vi "main 0.9.6.testing.vi"() -> ()   [LabVIEW 2015]
uses:
  subvi/PHOIBOS/DEFINITIONS/DEF_dev_state.ctl
  subvi/PHOIBOS/DEFINITIONS/DEF_dev_type.ctl
  <vilib>/Analysis/1siggen.llb/Ramp Pattern by Samples.vi
  <vilib>/DAQmx/read.llb/DAQmx Read (Digital Bool 1Line 1Point).vi
  <vilib>/Utility/file.llb/Write Delimited Spreadsheet (DBL).vi
  <vilib>/Utility/file.llb/Read Delimited Spreadsheet (string).vi
  <vilib>/DAQmx/create/channels.llb/DAQmx Create Channel (DI-Digital Input).vi
  <vilib>/DAQmx/miscellaneous.llb/DAQmx Fill In Error Info.vi
  subvi/Newport ESP301/Newport ESP301.lvlib
  subvi/sp_manip.llb/sp_manip_lib.lvlib
  subvi/sp_manip.llb/tcp_gateway.lvlib
  <vilib>/Analysis/NI_AALBase.lvlib
panel:
  in  "Enable Chopping":bool
  out "Pump Laser":bool
  out "Pics L":i32
  out "Pics NL":i32
  out "sideimg 2":dbl[][](graph)
  in  "Frame trigger \n(High Performance and QE only)":u16=1
  in  "Operating mode\nHP & QE / HS & DiCam Pro":u32
  out "Waveform Chart":dbl(graph)
  out "G2 X":cluster{dbl[], "Ramp Pattern":dbl[]}(graph)={array[344 elements], "Ramp Pattern"=[5593.0, 5541.0, 5578.0, 5573.0, 5542.0, 5582.0, 5523.0, 5570.0, 5578.0, 5560.0, 5581.0, 5542.0, 5577.0, 5517.0, 5599.0, 5558.0, 5549.0, 5571.0, 5527.0, 5574.0, 5565.0, 5561.0, 5570.0, 5531.0, 5576.0, 5531.0, 5576.0, 5554.0, 5523.0, 5573.0, 5536.0, 5555.0, 5539.0, 5549.0, 5543.0, 5541.0, 5581.0, 5523.0, 5548.0, 5528.0, 5558.0, 5565.0, 5537.0, 5556.0, 5521.0, 5538.0, 5549.0, 5532.0, 5562.0, 5512.0, 5555.0, 5549.0, 5536.0, 5542.0, 5511.0, 5567.0, 5526.0, 5549.0, 5545.0, 5543.0, 5562.0, 5518.0, 5561.0, 5490.0, 5542.0, 5522.0, 5529.0, 5542.0, 5521.0, 5556.0, 5511.0, 5541.0, 5534.0, 5512.0, 5569.0, 5525.0, 5547.0, 5507.0, 5533.0, 5533.0, 5501.0, 5555.0, 5497.0, 5517.0, 5526.0, 5519.0, 5565.0, 5503.0, 5548.0, 5496.0, 5544.0, 5523.0, 5534.0, 5533.0, 5501.0, 5529.0, 5494.0, 5523.0, 5526.0, 5519.0, 5539.0, 5493.0, 5508.0, 5532.0, 5504.0, 5546.0, 5540.0, 5550.0, 5488.0, 5556.0, 5535.0, 5510.0, 5535.0, 5515.0, 5543.0, 5475.0, 5538.0, 5528.0, 5504.0, 5523.0, 5502.0, 5535.0, 5473.0, 5503.0, 5501.0, 5531.0, 5525.0, 5490.0, 5524.0, 5484.0, 5520.0, 5506.0, 5492.0, 5516.0, 5477.0, 5511.0, 5487.0, 5509.0, 5496.0, 5467.0, 5538.0, 5494.0, 5512.0, 5497.0, 5498.0, 5526.0, 5482.0, 5506.0, 5466.0, 5522.0, 5489.0, 5512.0, 5518.0, 5475.0, 5547.0, 5480.0, 5569.0, 5504.0, 5485.0, 5528.0, 5506.0, 5529.0, 5468.0, 5524.0, 5507.0, 5518.0, 5511.0, 5471.0, 5525.0, 5480.0, 5482.0, 5510.0, 5506.0, 5522.0, 5475.0, 5540.0, 5477.0, 5511.0, 5514.0, 5500.0, 5497.0, 5484.0, 5536.0, 5476.0, 5485.0, 5527.0, 5509.0, 5529.0, 5495.0, 5504.0, 5496.0, 5519.0, 5512.0, 5469.0, 5506.0, 5465.0, 5502.0, 5481.0, 5508.0, 5519.0, 5499.0, 5515.0, 5476.0, 5496.0, 5502.0, 5499.0, 5494.0, 5477.0, 5541.0, 5477.0, 5512.0, 5497.0, 5472.0, 5511.0, 5471.0, 5503.0, 5507.0, 5504.0, 5477.0, 5479.0, 5508.0, 5481.0, 5522.0, 5517.0, 5516.0, 5505.0, 5502.0, 5491.0, 5481.0, 5512.0, 5484.0, 5500.0, 5478.0, 5493.0, 5529.0, 5492.0, 5518.0, 5471.0, 5518.0, 5490.0, 5513.0, 5497.0, 5488.0, 5517.0, 5477.0, 5524.0, 5464.0, 5495.0, 5514.0, 5495.0, 5522.0, 5477.0, 5490.0, 5535.0, 5489.0, 5491.0, 5491.0, 5515.0, 5473.0, 5504.0, 5505.0, 5515.0, 5510.0, 5473.0, 5521.0, 5475.0, 5537.0, 5499.0, 5505.0, 5509.0, 5460.0, 5509.0, 5473.0, 5489.0, 5500.0, 5464.0, 5522.0, 5471.0, 5528.0, 5475.0, 5502.0, 5494.0, 5511.0, 5516.0, 5486.0, 5528.0, 5471.0, 5492.0, 5477.0, 5491.0, 5531.0, 5486.0, 5549.0, 5498.0, 5524.0, 5482.0, 5495.0, 5505.0, 5476.0, 5512.0, 5444.0, 5512.0, 5498.0, 5471.0, 5489.0, 5462.0, 5502.0, 5459.0, 5503.0, 5489.0, 5493.0, 5498.0, 5461.0, 5505.0, 5495.0, 5503.0, 5459.0, 5501.0, 5515.0, 5459.0, 5510.0, 5469.0, 5504.0, 5499.0, 5505.0, 5524.0, 5477.0, 5527.0, 5477.0, 5475.0, 5495.0, 5482.0, 5514.0, 5481.0, 5499.0, 5481.0, 5482.0, 5498.0, 5460.0, 5469.0, 5471.0, 5519.0, 5495.0, 5485.0]}
  in  "reset every n pics":bool
  in  "pics2avg":i32=50
  in  "abort acq.":bool
  out "G2 Y":cluster{dbl[], "Ramp Pattern":dbl[]}(graph)={[5738.0, 5692.0, 5562.0, 5630.0, 5633.0, 5616.0, 5523.0, 5622.0, 5406.0, 5598.0, 5416.0, 5403.0, 5579.0, 5325.0, 5504.0, 5402.0, 5538.0, 5568.0, 5460.0, 5494.0, 5367.0, 5597.0, 5434.0, 5448.0, 5339.0, 5434.0, 5460.0, 5482.0, 5646.0, 5720.0, 5704.0, 5628.0, 5672.0, 5511.0, 5420.0, 5539.0, 5543.0, 5421.0, 5486.0, 5508.0, 5537.0, 5586.0, 5460.0, 5547.0, 5433.0, 5488.0, 5552.0, 5538.0, 5528.0, 5482.0, 5406.0, 5458.0, 5644.0, 5485.0, 5443.0, 5485.0, 5385.0, 5413.0, 5472.0, 5571.0, 5640.0, 5602.0, 5462.0, 5477.0, 5408.0, 5396.0, 5445.0, 5638.0, 5383.0, 5571.0, 5372.0, 5519.0, 5426.0, 5462.0, 5481.0, 5626.0, 5326.0, 5458.0, 5471.0, 5366.0, 5394.0, 5363.0, 5551.0, 5596.0, 5452.0, 5470.0, 5600.0, 5533.0, 5573.0, 5544.0, 5671.0, 5595.0, 5423.0, 5550.0, 5557.0, 5416.0, 5404.0, 5478.0, 5448.0, 5512.0, 5505.0, 5575.0, 5434.0, 5436.0, 5600.0, 5487.0, 5607.0, 5463.0, 5606.0, 5540.0, 5521.0, 5581.0, 5472.0, 5555.0, 5576.0, 5612.0, 5529.0, 5473.0, 5454.0, 5455.0, 5500.0, 5650.0, 5451.0, 5445.0, 5423.0, 5376.0, 5389.0, 5491.0, 5536.0, 5525.0, 5440.0, 5707.0, 5414.0, 5532.0, 5400.0, 5668.0, 5706.0, 5515.0, 5431.0, 5400.0, 5439.0, 5471.0, 5627.0, 5691.0, 5569.0, 5718.0, 5614.0, 5523.0, 5436.0, 5432.0, 5419.0, 5516.0, 5469.0, 5467.0, 5530.0, 5598.0, 5501.0, 5476.0, 5457.0, 5460.0, 5606.0, 5456.0, 5429.0, 5586.0, 5504.0, 5546.0, 5516.0, 5466.0, 5650.0, 5593.0, 5605.0, 5515.0, 5414.0, 5623.0, 5581.0, 5651.0, 5574.0, 5519.0, 5672.0, 5621.0, 5496.0, 5382.0, 5496.0, 5620.0, 5542.0, 5422.0, 5492.0, 5515.0, 5549.0, 5402.0, 5472.0, 5547.0, 5515.0, 5641.0, 5451.0, 5667.0, 5622.0, 5511.0, 5506.0, 5608.0, 5647.0, 5584.0, 5714.0, 5490.0, 5534.0, 5463.0, 5566.0, 5573.0, 5570.0, 5582.0, 5613.0, 5504.0, 5550.0, 5594.0, 5576.0, 5677.0, 5675.0, 5681.0, 5681.0, 5434.0, 5434.0, 5405.0, 5473.0, 5522.0, 5427.0, 5533.0, 5582.0, 5427.0, 5529.0, 5548.0, 5341.0, 5521.0, 5539.0, 5435.0, 5457.0, 5511.0, 5406.0, 5412.0, 5620.0, 5609.0, 5609.0, 5469.0, 5577.0, 5661.0, 5673.0, 5518.0, 5463.0, 5562.0, 5723.0, 5719.0, 5487.0, 5485.0, 5683.0, 5501.0, 5604.0, 5328.0], "Ramp Pattern"=[0.0, 1.003921568627451, 2.007843137254902, 3.011764705882353, 4.015686274509804, 5.019607843137255, 6.023529411764706, 7.027450980392157, 8.031372549019608, 9.035294117647059, 10.03921568627451, 11.04313725490196, 12.047058823529412, 13.050980392156863, 14.054901960784314, 15.058823529411764, 16.062745098039215, 17.066666666666666, 18.070588235294117, 19.07450980392157, 20.07843137254902, 21.08235294117647, 22.08627450980392, 23.090196078431372, 24.094117647058823, 25.098039215686274, 26.101960784313725, 27.105882352941176, 28.109803921568627, 29.113725490196078, 30.11764705882353, 31.12156862745098, 32.12549019607843, 33.129411764705885, 34.13333333333333, 35.13725490196079, 36.141176470588235, 37.14509803921569, 38.14901960784314, 39.15294117647059, 40.15686274509804, 41.16078431372549, 42.16470588235294, 43.168627450980395, 44.17254901960784, 45.1764705882353, 46.180392156862744, 47.1843137254902, 48.188235294117646, 49.1921568627451, 50.19607843137255, 51.2, 52.20392156862745, 53.207843137254905, 54.21176470588235, 55.21568627450981, 56.219607843137254, 57.22352941176471, 58.227450980392156, 59.23137254901961, 60.23529411764706, 61.23921568627451, 62.24313725490196, 63.247058823529414, 64.25098039215686, 65.25490196078431, 66.25882352941177, 67.26274509803922, 68.26666666666667, 69.27058823529411, 70.27450980392157, 71.27843137254902, 72.28235294117647, 73.28627450980392, 74.29019607843138, 75.29411764705883, 76.29803921568627, 77.30196078431372, 78.30588235294118, 79.30980392156863, 80.31372549019608, 81.31764705882352, 82.32156862745099, 83.32549019607843, 84.32941176470588, 85.33333333333333, 86.33725490196079, 87.34117647058824, 88.34509803921569, 89.34901960784313, 90.3529411764706, 91.35686274509804, 92.36078431372549, 93.36470588235294, 94.3686274509804, 95.37254901960785, 96.37647058823529, 97.38039215686274, 98.3843137254902, 99.38823529411765, 100.3921568627451, 101.39607843137254, 102.4, 103.40392156862745, 104.4078431372549, 105.41176470588235, 106.41568627450981, 107.41960784313726, 108.4235294117647, 109.42745098039215, 110.43137254901961, 111.43529411764706, 112.43921568627451, 113.44313725490196, 114.44705882352942, 115.45098039215686, 116.45490196078431, 117.45882352941176, 118.46274509803922, 119.46666666666667, 120.47058823529412, 121.47450980392156, 122.47843137254903, 123.48235294117647, 124.48627450980392, 125.49019607843137, 126.49411764705883, 127.49803921568628, 128.50196078431372, 129.50588235294117, 130.50980392156862, 131.51372549019607, 132.51764705882354, 133.521568627451, 134.52549019607844, 135.52941176470588, 136.53333333333333, 137.53725490196078, 138.54117647058823, 139.54509803921567, 140.54901960784315, 141.5529411764706, 142.55686274509804, 143.5607843137255, 144.56470588235294, 145.5686274509804, 146.57254901960783, 147.57647058823528, 148.58039215686276, 149.5843137254902, 150.58823529411765, 151.5921568627451, 152.59607843137255, 153.6, 154.60392156862744, 155.6078431372549, 156.61176470588236, 157.6156862745098, 158.61960784313726, 159.6235294117647, 160.62745098039215, 161.6313725490196, 162.63529411764705, 163.6392156862745, 164.64313725490197, 165.64705882352942, 166.65098039215687, 167.65490196078431, 168.65882352941176, 169.6627450980392, 170.66666666666666, 171.6705882352941, 172.67450980392158, 173.67843137254903, 174.68235294117648, 175.68627450980392, 176.69019607843137, 177.69411764705882, 178.69803921568626, 179.7019607843137, 180.7058823529412, 181.70980392156864, 182.71372549019608, 183.71764705882353, 184.72156862745098, 185.72549019607843, 186.72941176470587, 187.73333333333332, 188.7372549019608, 189.74117647058824, 190.7450980392157, 191.74901960784314, 192.75294117647059, 193.75686274509803, 194.76078431372548, 195.76470588235293, 196.7686274509804, 197.77254901960785, 198.7764705882353, 199.78039215686275, 200.7843137254902, 201.78823529411764, 202.7921568627451, 203.79607843137254, 204.8, 205.80392156862746, 206.8078431372549, 207.81176470588235, 208.8156862745098, 209.81960784313725, 210.8235294117647, 211.82745098039214, 212.83137254901962, 213.83529411764707, 214.8392156862745, 215.84313725490196, 216.8470588235294, 217.85098039215686, 218.8549019607843, 219.85882352941175, 220.86274509803923, 221.86666666666667, 222.87058823529412, 223.87450980392157, 224.87843137254902, 225.88235294117646, 226.8862745098039, 227.89019607843136, 228.89411764705883, 229.89803921568628, 230.90196078431373, 231.90588235294118, 232.90980392156862, 233.91372549019607, 234.91764705882352, 235.92156862745097, 236.92549019607844, 237.9294117647059, 238.93333333333334, 239.93725490196078, 240.94117647058823, 241.94509803921568, 242.94901960784313, 243.95294117647057, 244.95686274509805, 245.9607843137255, 246.96470588235294, 247.9686274509804, 248.97254901960784, 249.9764705882353, 250.98039215686273, 251.98431372549018, 252.98823529411766, 253.9921568627451, 254.99607843137255, 256.0]}
  out "ETA":timestamp=timestamp(3543843884.995538 s since 1904-01-01) format="%<%H:%M:%S>T"
  out "acq. imgs":i32=30
  out "snap_prog":dbl(slide)=1.0 scale=0.0..1.0
  in  "BasePath":path=path "C:/Users/femtolab_admin/Desktop"
  in  "cam_liveavg":bool caption="live average"
  out "cam_fps":dbl=20.079713544692744 caption="FPS" format="%.1g"
  out "sideimg":dbl[][](graph)
  in  "RunNumber":u16=77
  out "sum":dbl=4126991.0 format="%#.2g"
  out "max":dbl=54.0
  out "mainimg":dbl[][](graph)
  out "ESP_con?":bool=TRUE caption="ESP301"
  out "phoib_con?":bool caption="PHOIBOS"
  out "manip_con?":bool caption="manipulator"
  out "cam_con?":bool caption="camera"
  in  "main_close":bool
  in  "Tab Control":T1(tab)
  in  "manip_deltas":dbl[](array[numeric])=[0.0, 0.0, 0.0, 0.0, 10.0, 0.0] caption="delta" format="%#.5g"
  in  "aq.mode":enum32{"Radio Selection 1", "Radio Selection 2"}(radio)=enum."Radio Selection 2"
  in  "dark avg":i32=100
  in  "averages":i32=30 caption="N"
  in  "ESP_delta":dbl caption="relative [mm]"
  in  "ESP_-":bool
  in  "ESP_+":bool
  in  "ESP_go":bool
  in  "ESP_dest_t":dbl=250.17307139859977 caption="[fs]"
  in  "ESP_dest":dbl=31.304 caption="[mm]"
  in  "ESP_set_t0":bool
  in  "phoib_I_6s":dbl=3200.0
  in  "phoib_I_5s":dbl=1650.0
  in  "phoib_I_4s":dbl=4.558
  in  "phoib_I_3s":dbl=-7.0
  in  "phoib_I_2s":dbl=20.0
  in  "phoib_I_1s":dbl=22.0
  in  "phoib_standby":bool
  in  "phoib_set":bool
  out "phoib_I_6":dbl caption="Screen Voltage"
  out "phoib_I_5":dbl caption="Detctor Voltage"
  out "phoib_I_4":dbl caption="Work Function"
  out "phoib_I_3":dbl caption="Coil Current"
  out "phoib_I_2":dbl caption="Pass Energy"
  out "phoib_I_1":dbl caption="Kinetic Energy"
  out "Saved Positions":string[][](table)=[["ertwertwert", "-2.299945", "-2.030214", "38.900024", "50.000762", "0.000887", "-97.998082"], ["uztgugt", "-14.999451", "-13.638894", "442.380066", "13.998380", "-1.893758", "-76.305838"], ["asdf", "-14.999451", "-13.638894", "442.380066", "13.998380", "-1.893758", "-76.305838"], ["test3", "-14.999451", "-13.638894", "441.380066", "13.998380", "-1.893758", "-76.305838"]]
  in  "Save Pos":bool
  in  "Load":bool
  in  "Delete":bool
  in  "ManipRel +":bool
  in  "ManipRel -":bool
  in  "Move Abs":bool
  in  "stop manip":bool
  in  "dest":dbl[](array[numeric])=[-2.6172862113166087, -0.009888298846365134, 68.5008544921875, -46.36280498847848, 1.1073518432055398, -218.56360350415366] caption="destination" format="%#.5g"
  out "axis":string[](array[string])=["x", "y", "z", "polar", "tilt", "azimut"]
  out "pos":dbl[](array[numeric])=[-2.6172862113166087, -0.009888298846365134, 68.5008544921875, -46.363686276590336, 11.108982061941884, -218.56360350415366] caption="position" format="%.5f"
  in  "Mode":T2(ring)=enum."WideAngleMode"
  in  "VoltageRange":enum16{"3.5kV", "1.5kV", "400V", "100V", "10V"}(ring)=enum."400V"
  out "ESP_pos":dbl=31.4539 caption="Position"
  out "ESP_delay":dbl=1000.0251574040756 caption="Delay"
  out "ESP_t0":dbl=31.304 caption="Time Zero @"
  out "phoib_I_7":dbl caption="Conversion Voltage"
  in  "phoib_I_7s":dbl=-16.0
  in  "phoib_I_8s":dbl=0.0039
  in  "phoib_I_9s":dbl=0.0039
  out "phoib_I_8":dbl caption="FD1"
  out "phoib_I_9":dbl caption="FD2"
  in  "gain":bool
  in  "exposure [ms]":u32=1
  in  "binning":u16(ring)=2 items=["X 1", "X 2", "X 4", "X 8"]
  in  "cam_dark?":bool caption="subtract dark?"
  in  "cam_dark":bool
  in  "cam_saveimg":bool
  in  "e-size":u8
  in  "lower threshold":i32=-100
  in  "count?":bool
  in  "ROI Left":i32=1
  in  "ROI Right":i32=43
  in  "ROI Top":i32=1
  in  "ROI Bottom":i32=33
  out "moving?":bool[](array[boolean])
  in  "delscan_abort 2":bool
  in  "delscan_go 2":bool
  in  "delscan_finishIteration 2":bool
  out "del_ETA":timestamp=timestamp(3543843871.185777 s since 1904-01-01) format="%<%H:%M:%S>T"
  out "time / step":dbl=2.792118032773336
  out "duration [HH:MM:SS]":dbl=55.62603882380894 format="%<%H:%M:%S>t"
  out "disk [MB]":dbl=11.613000000000001
  out "RAM [MB]":dbl=2.765
  out "total steps":dbl=20.0
  out "delaypoints":dbl=5.0
  in  "generate delay table":bool
  in  "load delay table":bool
  in  "delay table [fs]":string[][](table)=[["-1000.000000"], ["-500.000000"], ["0.000000"], ["500.000000"], ["1000.000000"]]
  in  "delscan_iters":u32=4 caption="iterations"
  out "scangraph":T3(graph)
  in  "delscan_abort":bool
  out "delscan_progress":u32(slide)=5 scale=0.0..11.0
  in  "delscan_go":bool
  out "delscan_pos":dbl=31.453896228999998 caption="stage pos [mm]"
  in  "delscan_end":dbl=1000.0 caption="end [fs]"
  in  "delscan_stepsize":dbl=500.0 caption="stepsize [fs]"
  in  "delscan_start":dbl=-1000.0 caption="start [fs]"
  out "iteration":i32=5
  in  "delscan_finishIteration":bool
  in  "manip_scan_steps":u32=3
  in  "Optimize":bool
  in  "manip_scan_delta":dbl[](array[numeric])=[0.0, 0.0, 0.0, 0.0, 1.0, 0.0] caption="delta" format="%#.5g"
  out "delscan_progress 2":u32(slide)=2 scale=0.0..3.0
  in  "abort":bool
  in  "dev_bench":bool
  out "x/y":dbl
  out "1/x":dbl
  in  "stop":bool
  out "voltage out":dbl
  in  "manip_init":bool
  in  "manip_release":bool
  in  "phoib_init":bool
  in  "phoib_release":bool
  in  "ESP_init":bool
  in  "ESP_release":bool
  in  "ESP301 VISA":refnum<visa-resource-name>="COM8"
  in  "board number":i32
  in  "cam_init":bool
  in  "cam_release":bool
  out "cam_error":errorcluster
  out "phoib_error":errorcluster
  out "state":T4 items=["Off"=-1, "Standby"=0, "On"=1]
  in  "ESP Axis":i32=1 min=1 max=3
  out "error out":errorcluster
  out "error out 2":errorcluster={"status"=TRUE, "code"=1, "source"="TCP Write in sp_manip_lib.lvlib:sp_manip_disconnect.vi->main 0.9.1.vi"}
  # "0 = sequential\n1 = simultaneous"
  # "0 = internal\n1 = external rising\n2 = external falling"
  # "camera"
  # "analyzer"
  # "manipulator"
  # "aquisition"
  # "delay stage"
  # "Position"
  # "Destination"
  # "X\nY\nZ\npolar\ntilt\nazimut"
  # "camera"
  # "phoibos"
  # "ESP301"
  # "manipulator"
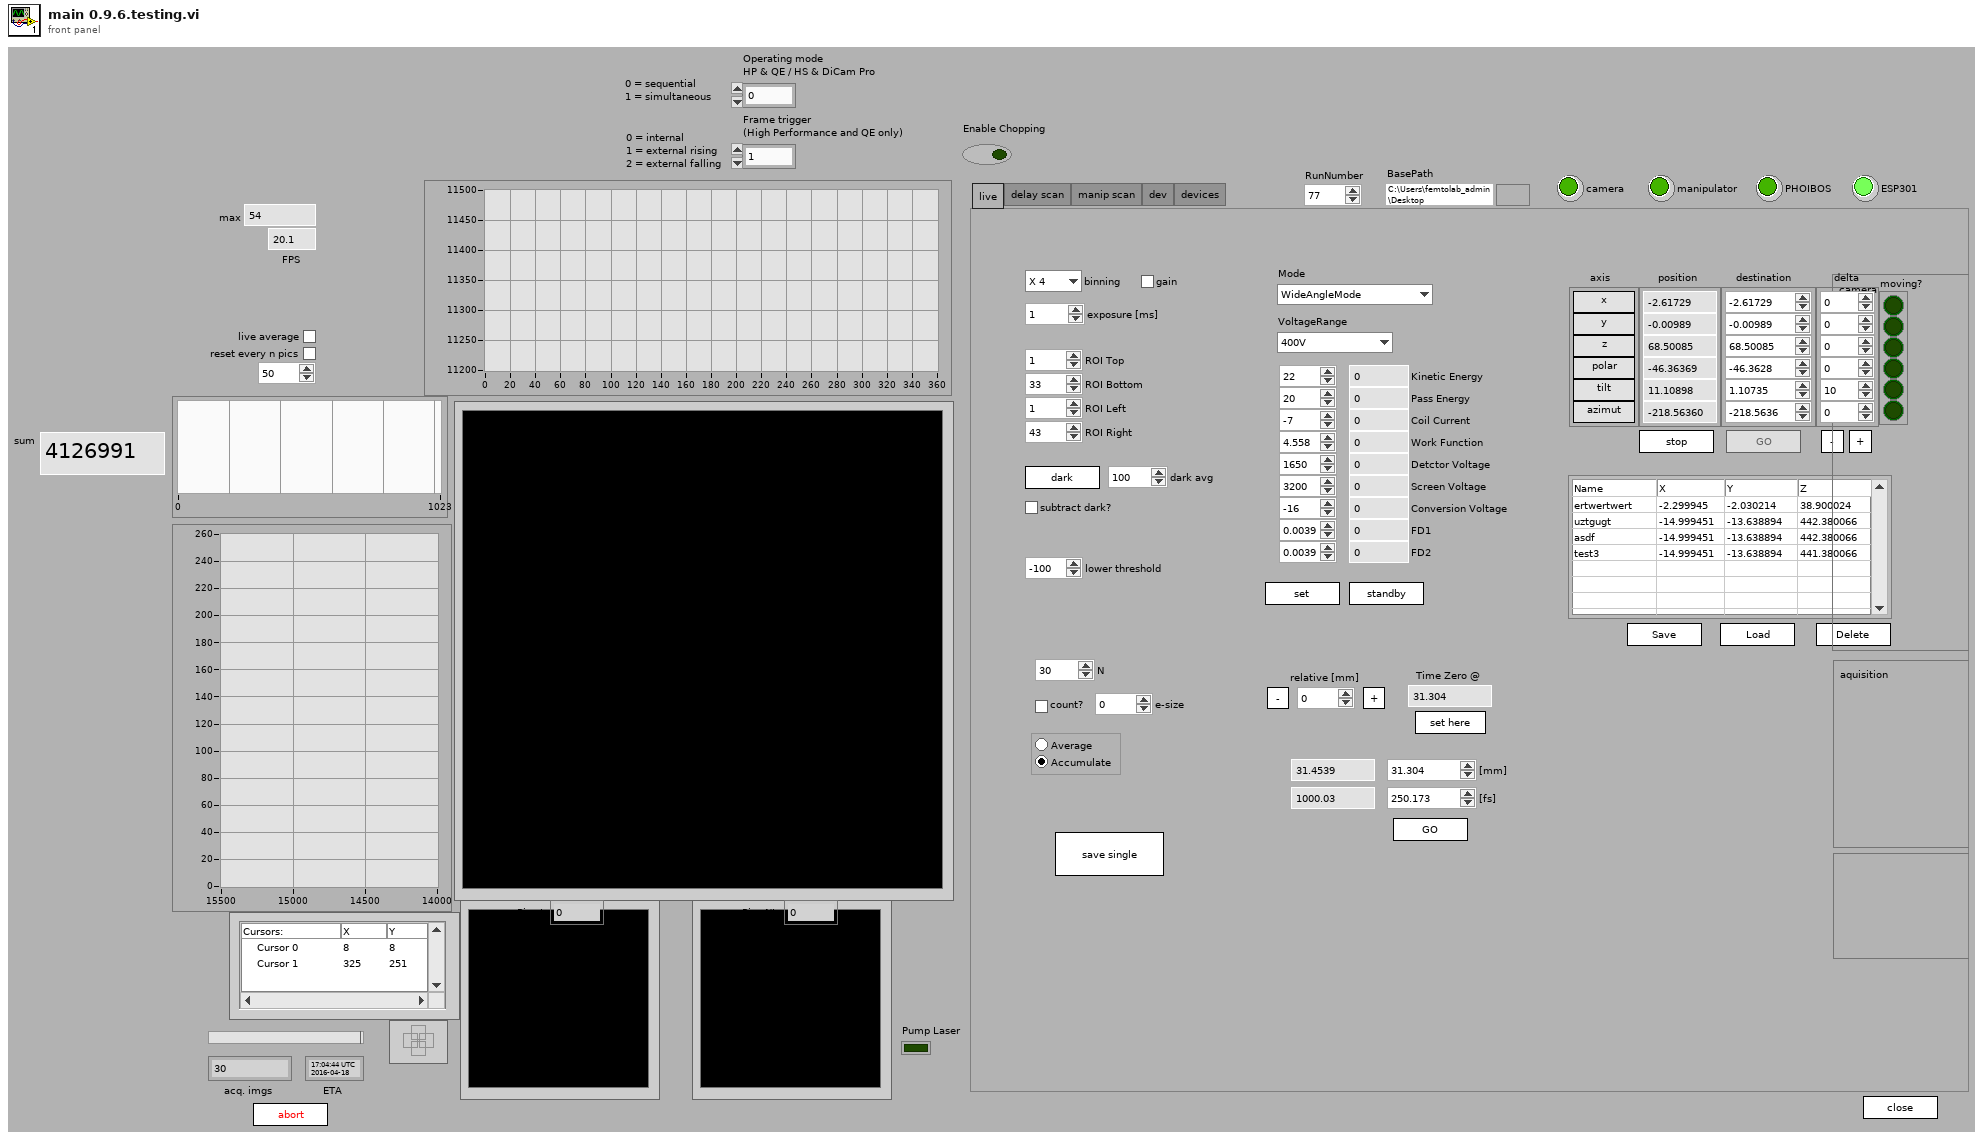
[diagram p1: front panel]
types:
  T1 = enum32{"live", "delay scan", "manip scan", "dev", "devices"}
  T2 = enum16{"HighMagnification", "MediumMagnification", "LowMagnification", "HighAngularDispersion", "MediumAngularDispersion", "LowAngularDispersion", "WideAngleMode", "LargeArea", "MediumArea", "SmallArea", "HighMagnification2", "SmallArea2", "ImagingMode"}
  T3 = cluster{"delay pointss [fs]":dbl[], "Intensity Chart":dbl[]}[]
  T4 = typedef "DEF_dev_state.ctl" = i32
  T5 = typedef "LVCursorListTypeDef.ctl" = cluster{"Name":string, "Color":u32, "Style":u8, "Point Style":u8, "Name Visible":bool, "Allow Drag":bool, "Cursor Mode":u32, "Plot":i32, "Index":i32, "Position":cluster{"X":dbl, "Y":dbl}, "X Scale":u32, "Y Scale":u32, "Watch Plots":i32[], "Watch All Plots":bool, "Plot Area":i32, "Label Offset":cluster{"X":dbl, "Y":dbl}}[]
  T6 = cluster{"delay pointss [fs]":dbl[], "Intensity Chart":dbl[]}
  T7 = cluster{"Camera type":u32, "Operating mode\nHP & QE / HS & DiCam Pro ":u32, "Frame trigger \n(High Performance and QE only)":u16, "Sequence trigger":u16, "Low Light\n(QE only)":bool, "Gain":bool, "Horzontal\nbinning":u16, "Vertical\nbinning ":u16, "ROI Left":i32, "ROI Right":i32, "ROI Top":i32, "ROI Bottom":i32}
  T8 = cluster{"Name":string, "Color":u32, "Style":u8, "Point Style":u8, "Name Visible":bool, "Allow Drag":bool, "Cursor Mode":u32, "Plot":i32, "Index":i32, "Position":cluster{"X":dbl, "Y":dbl}, "X Scale":u32, "Y Scale":u32, "Watch Plots":i32[], "Watch All Plots":bool, "Plot Area":i32, "Label Offset":cluster{"X":dbl, "Y":dbl}}
  T9 = cluster{"Axis_Name":string, "Axis_Type":string, "Axis_Position":dbl, "continous":bool, "moving":bool}[]
  T10 = typedef "DEF_dev_type.ctl" = enum32{"devA (analyzer)", "devD (detector)"}
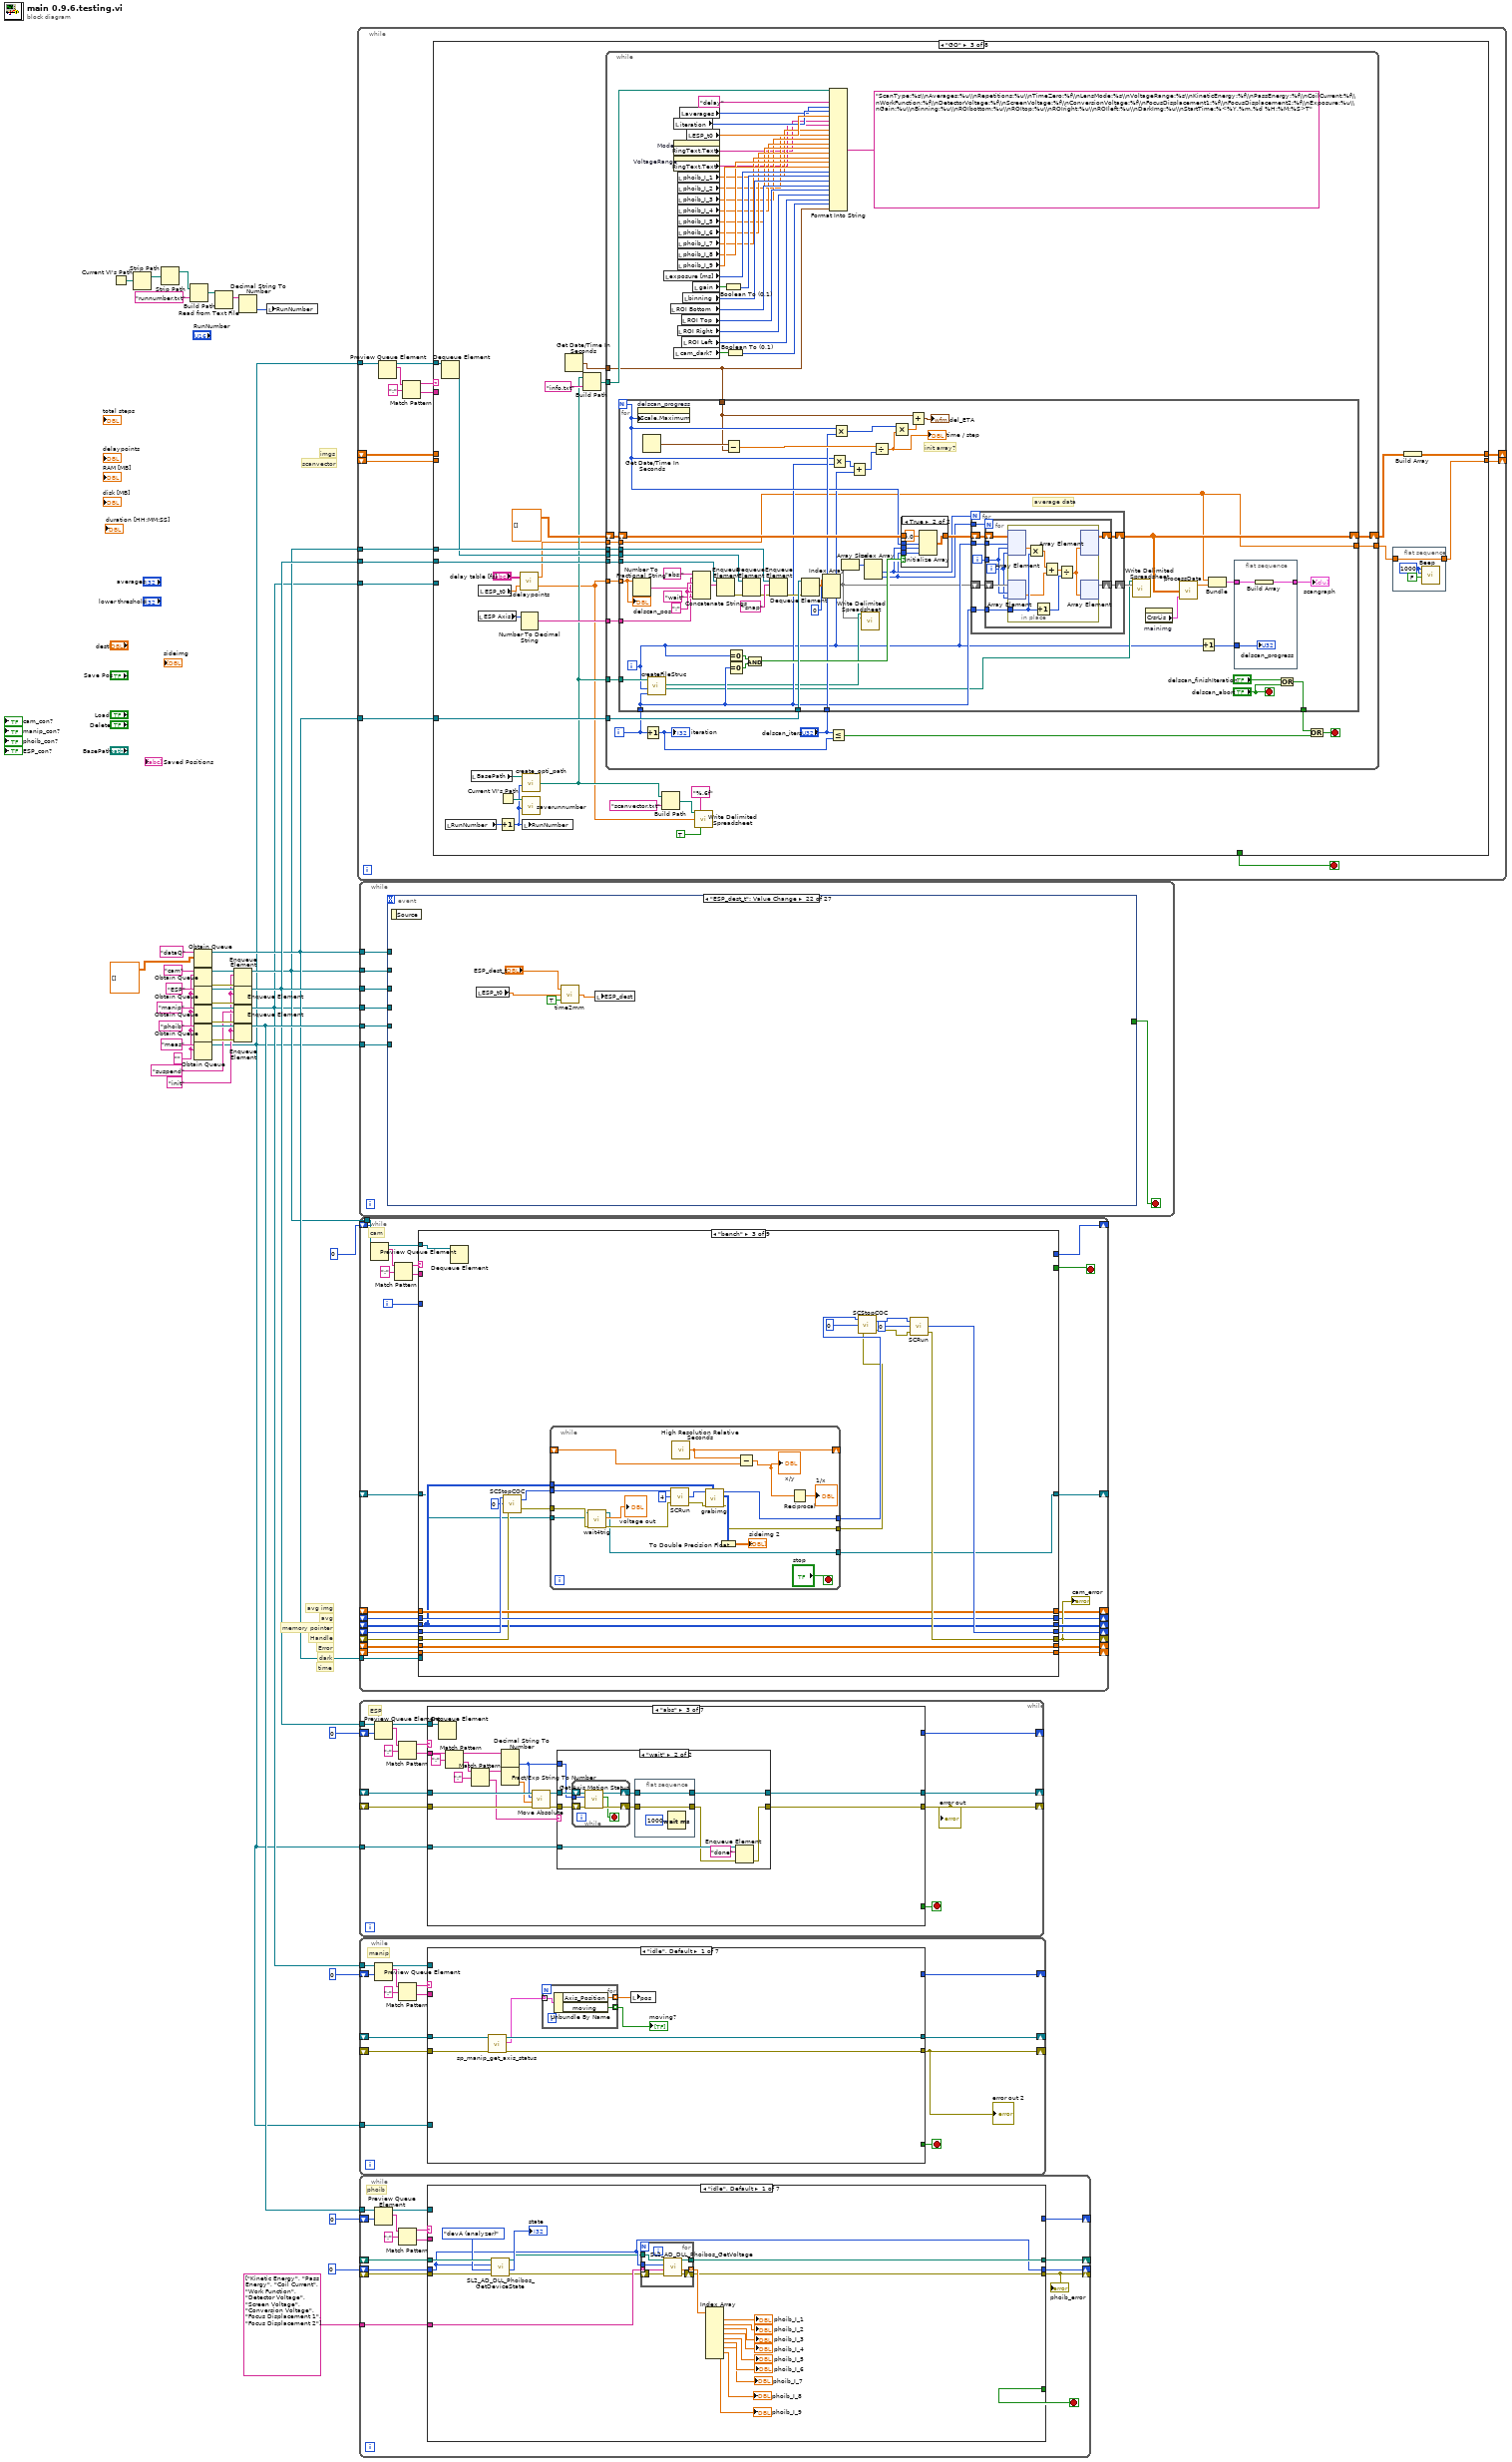
[diagram p0: block diagram]
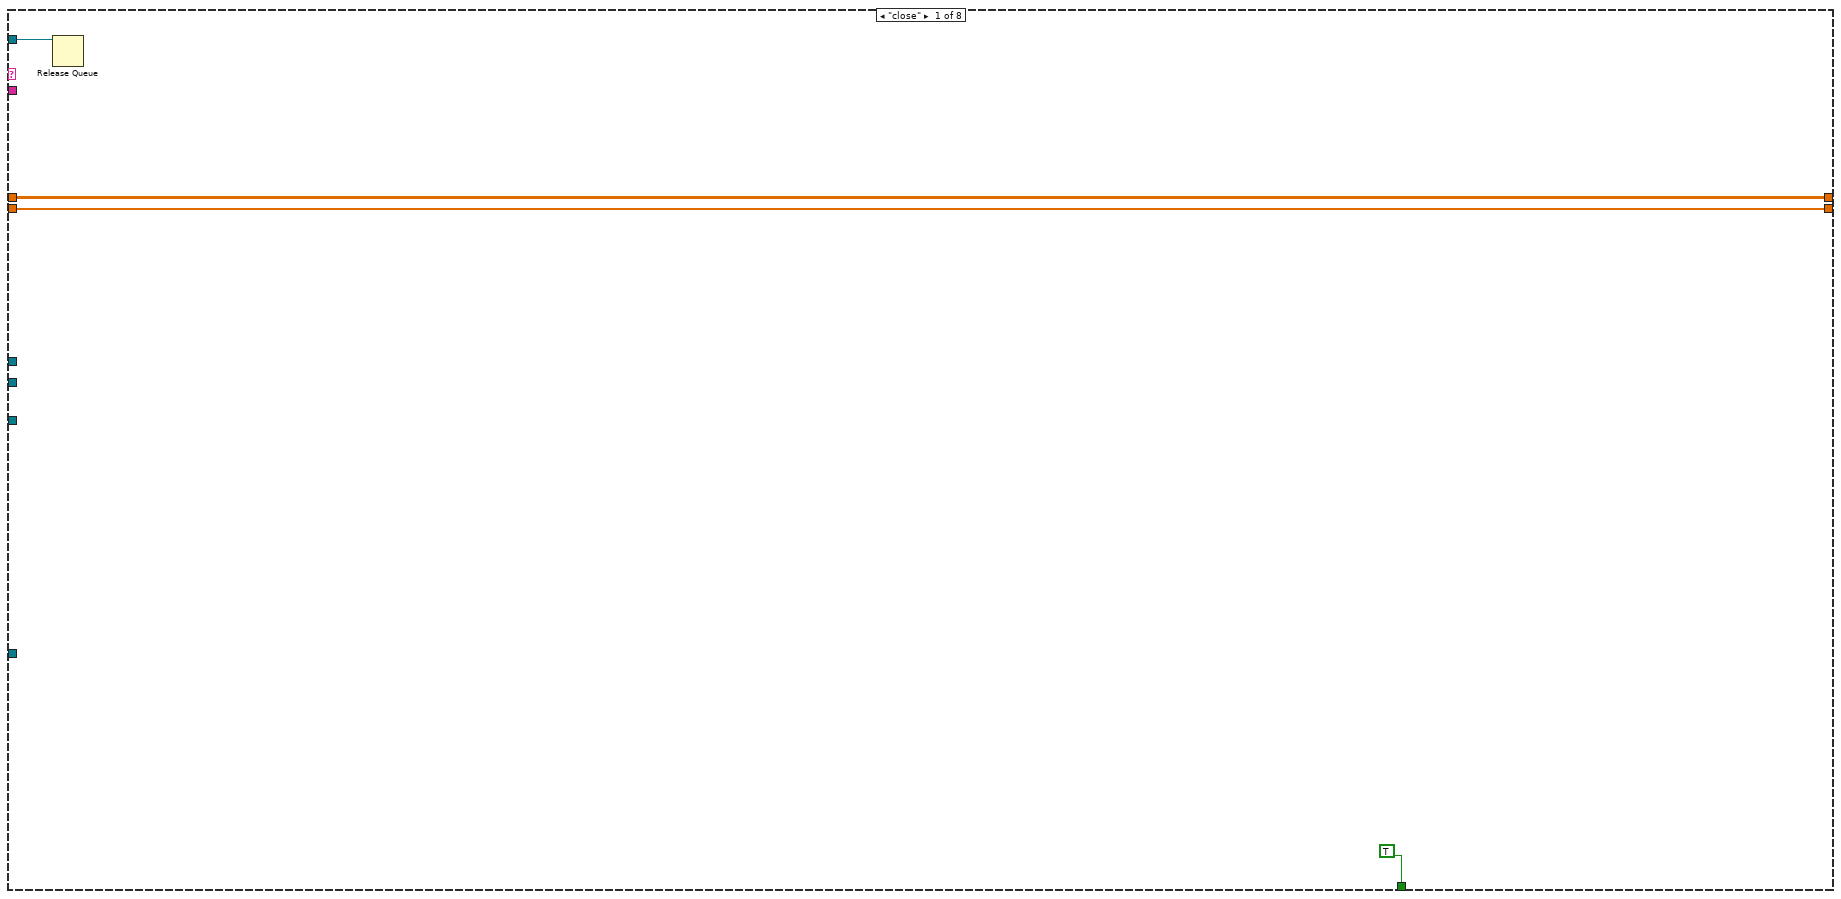
[diagram p2: hidden frame]
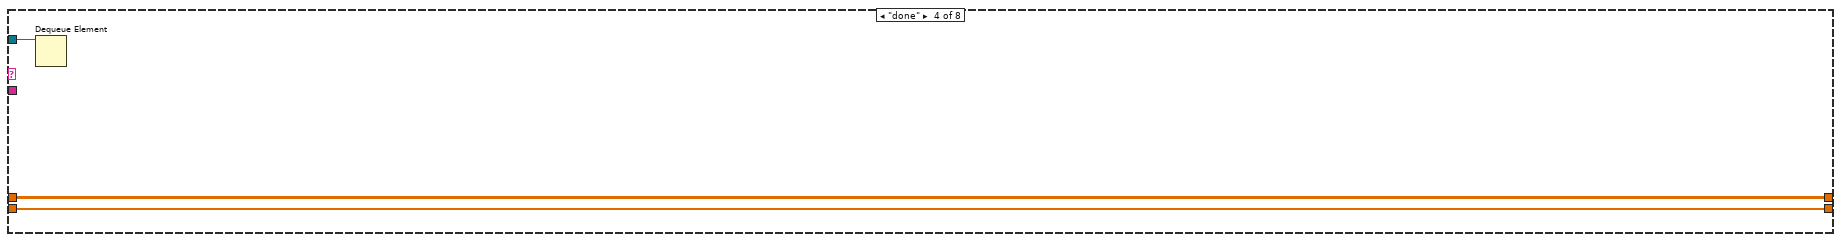
[diagram p5: hidden frame]
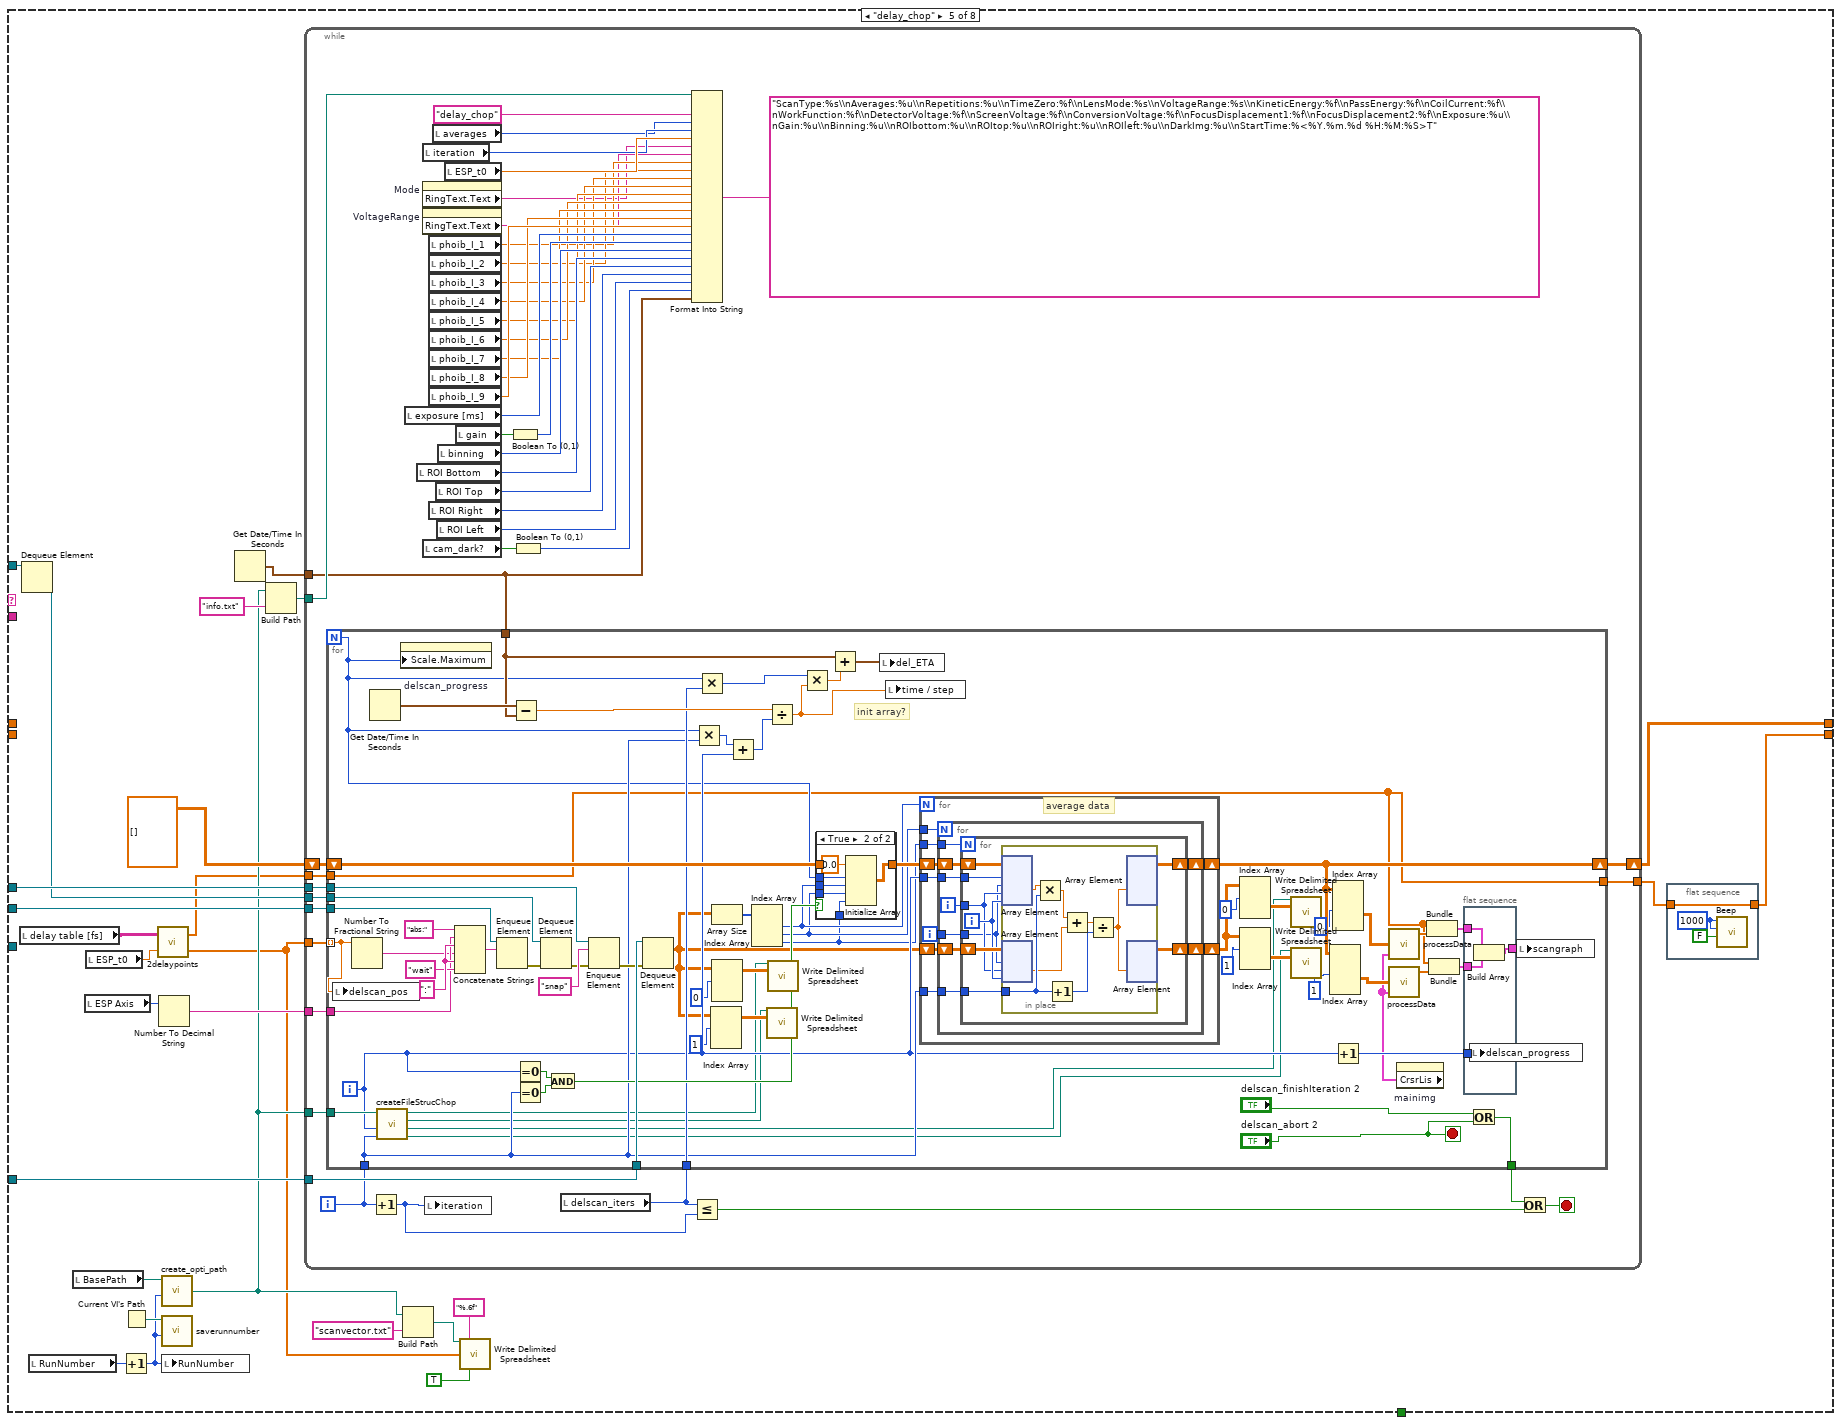
[diagram p6: hidden frame]
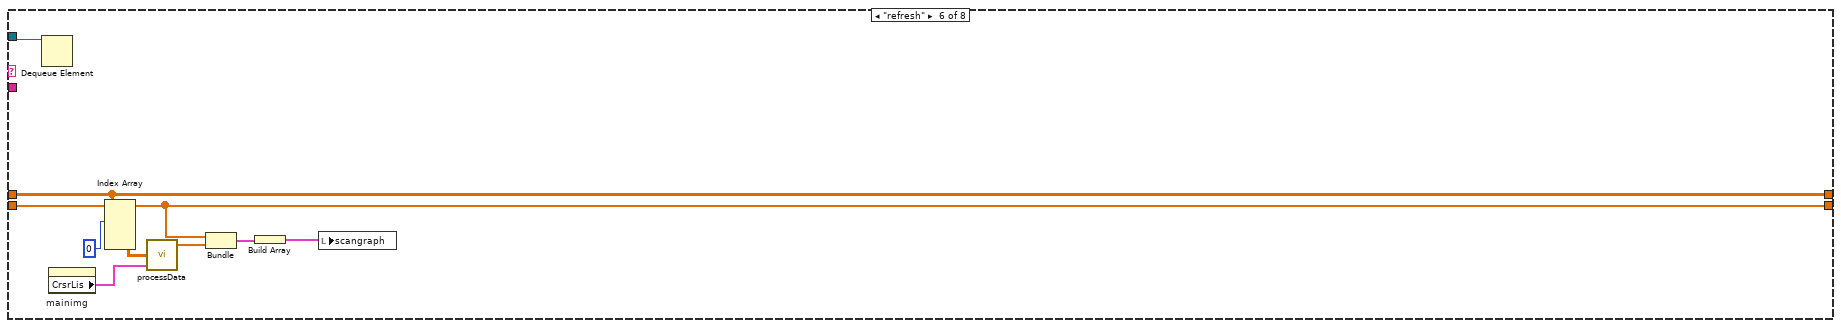
[diagram p8: hidden frame]
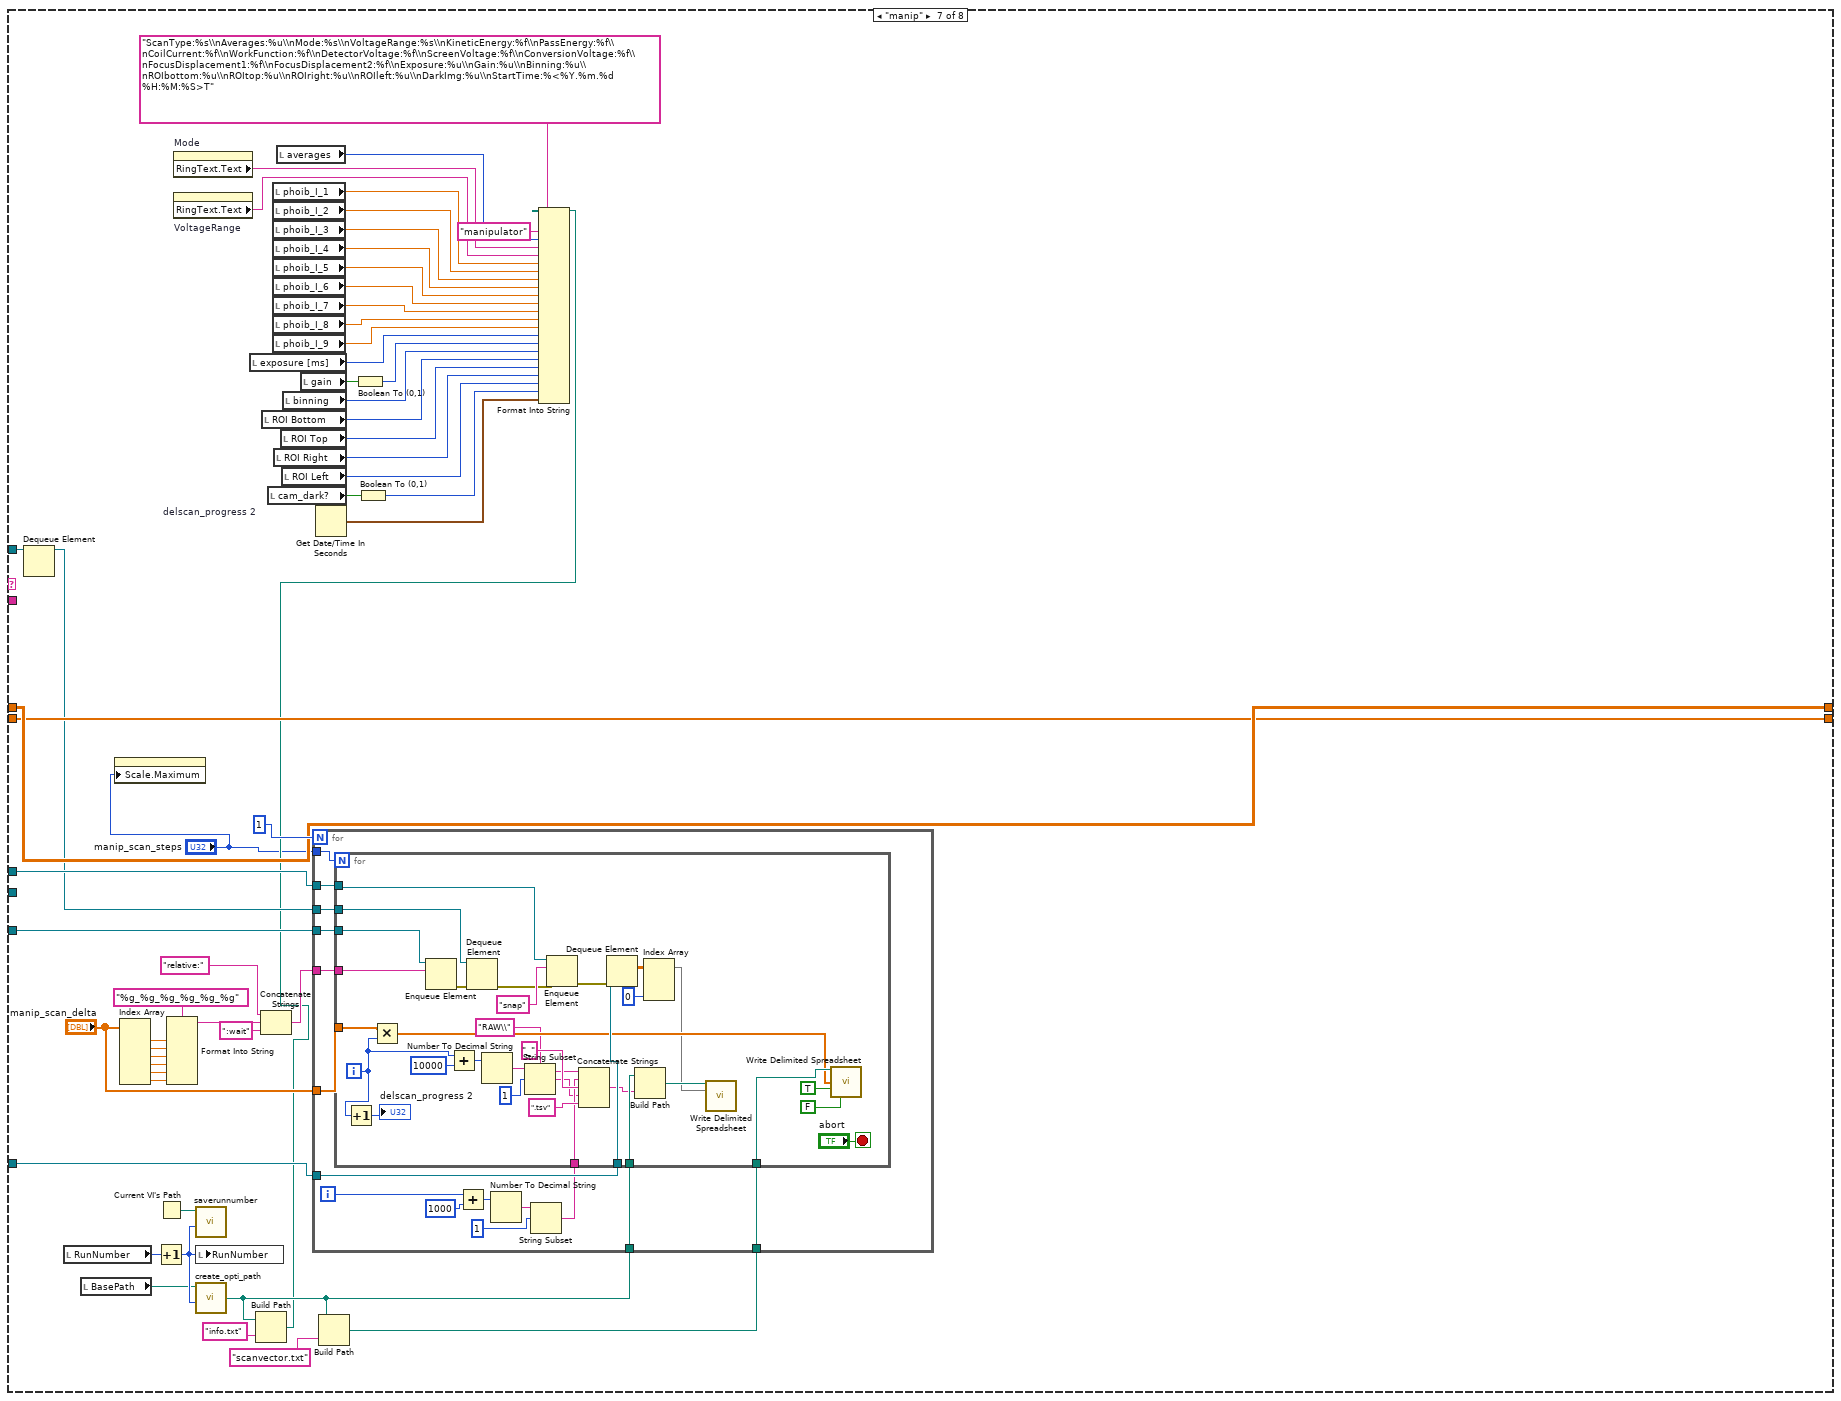
[diagram p9: hidden frame]
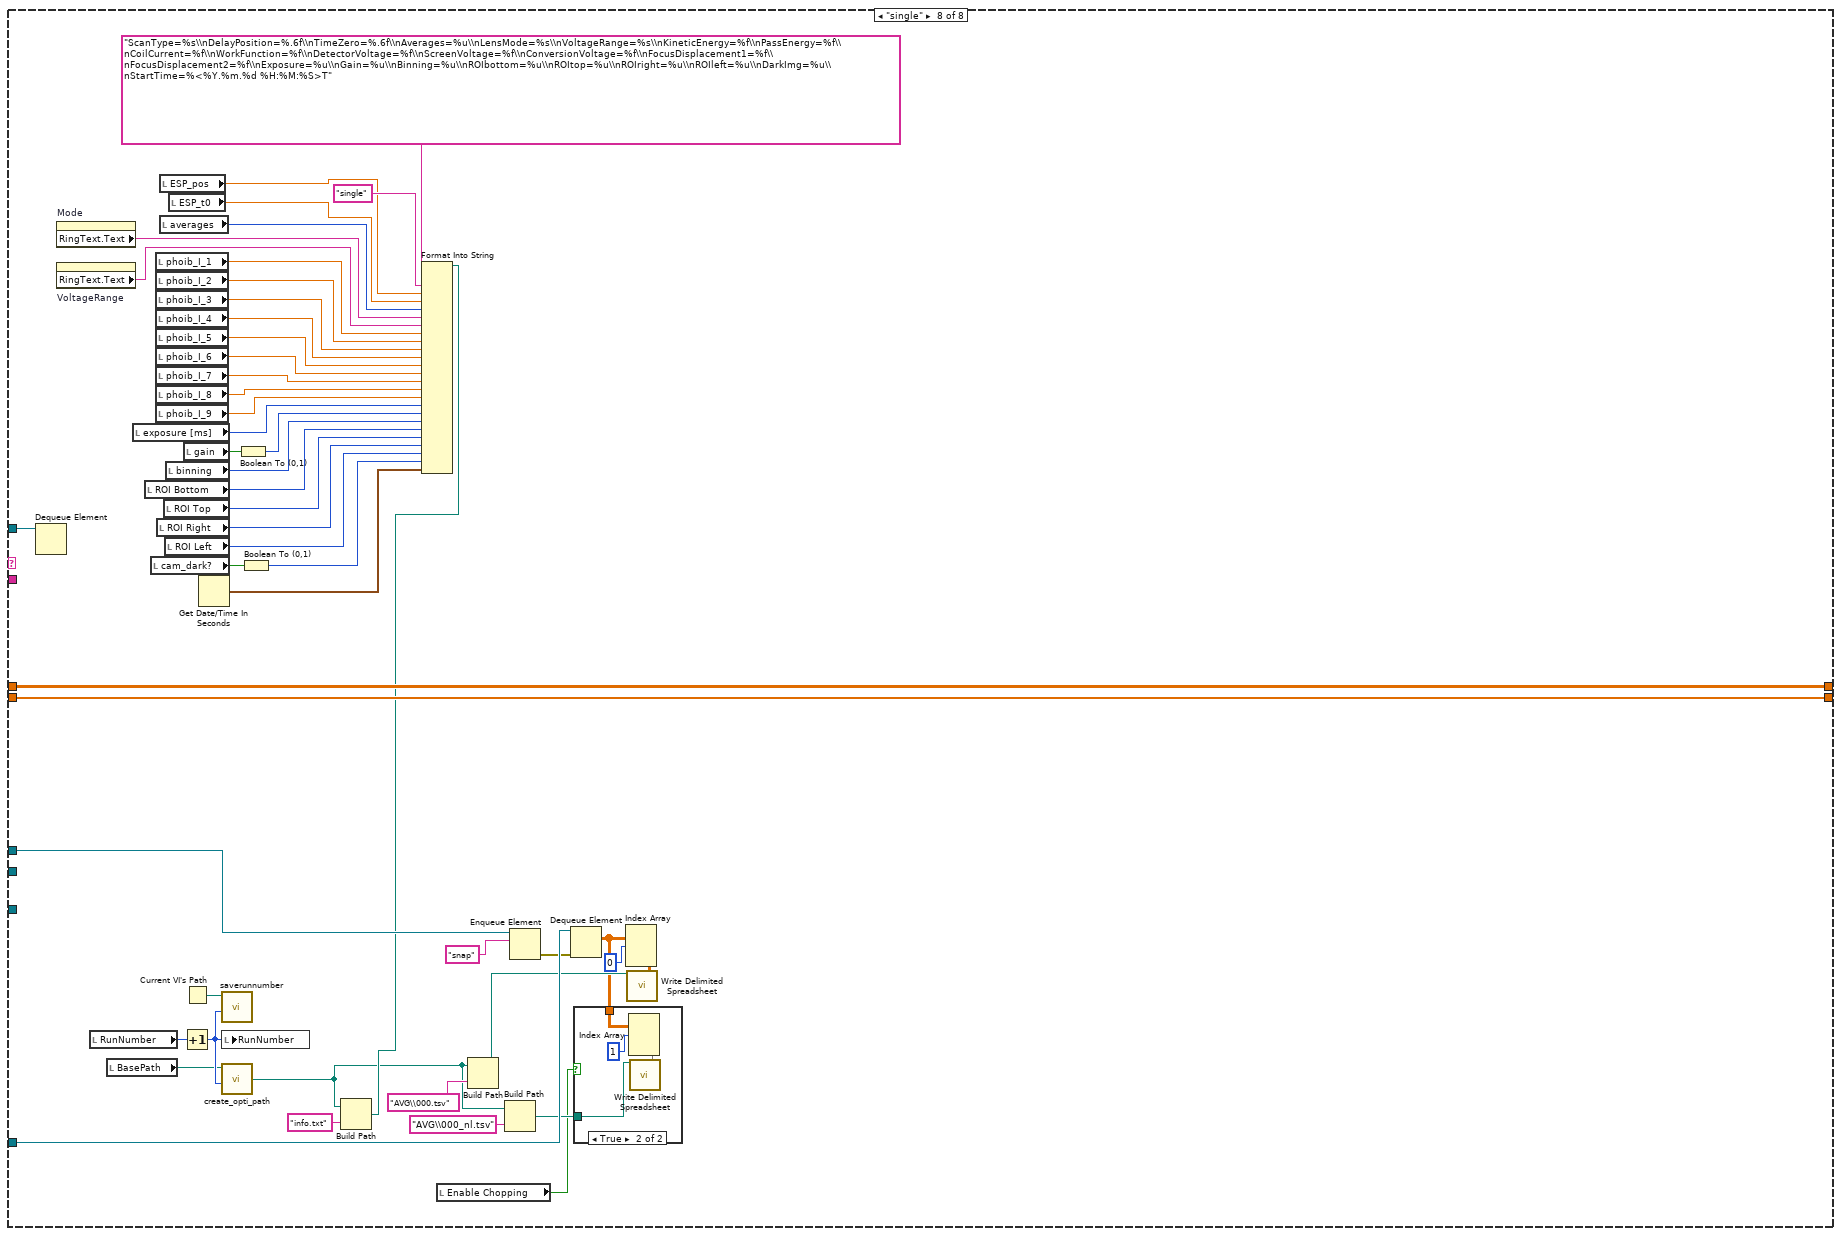
[diagram p10: hidden frame]
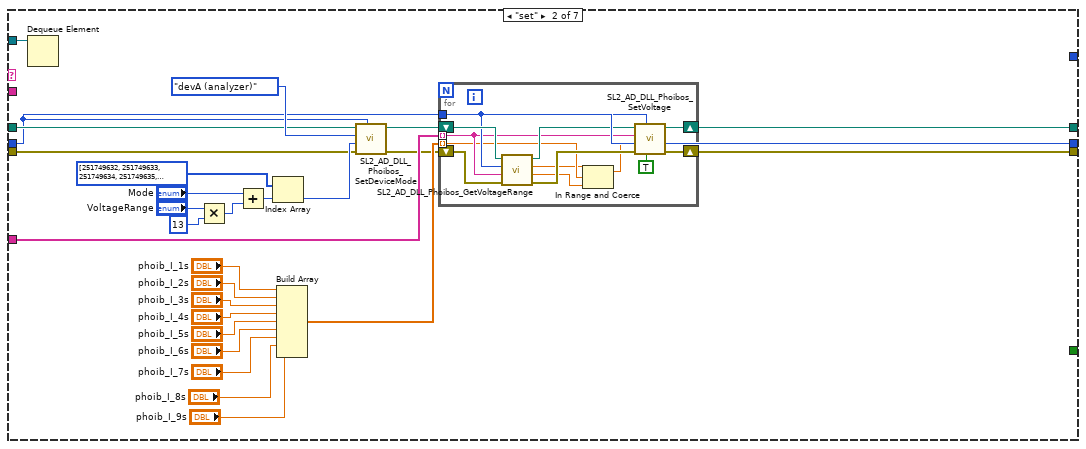
[diagram p12: hidden frame]
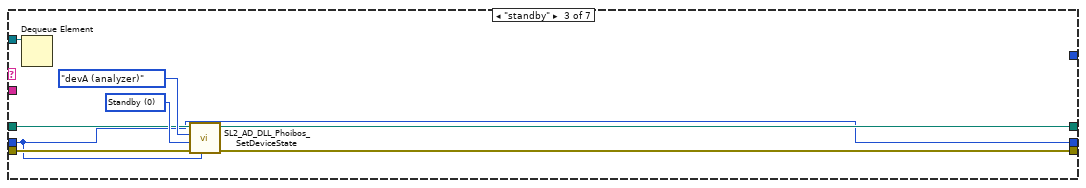
[diagram p13: hidden frame]
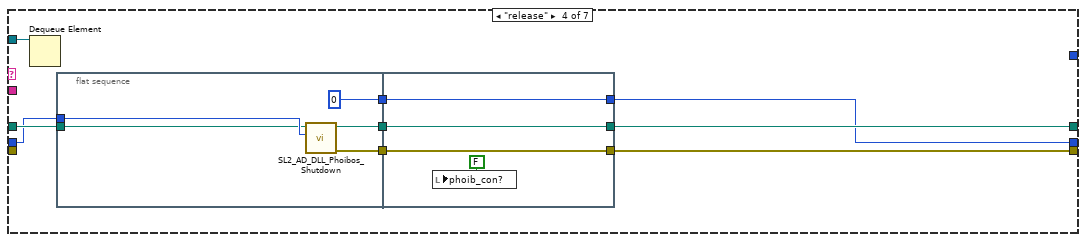
[diagram p14: hidden frame]
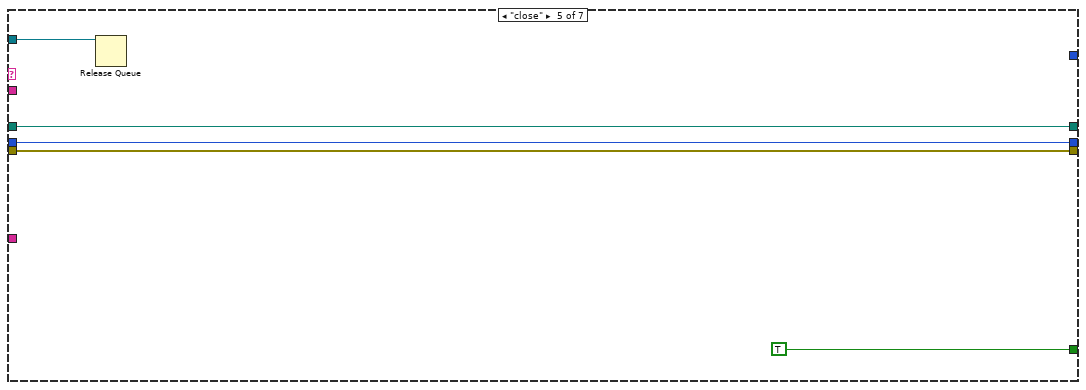
[diagram p15: hidden frame]
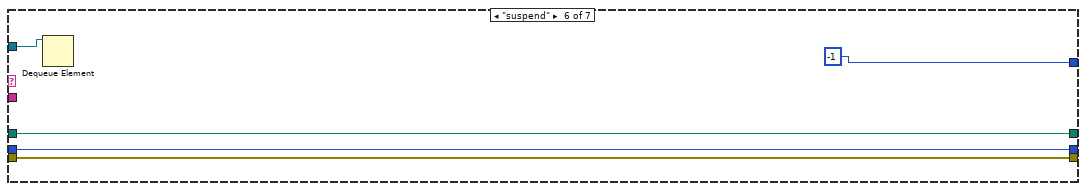
[diagram p16: hidden frame]
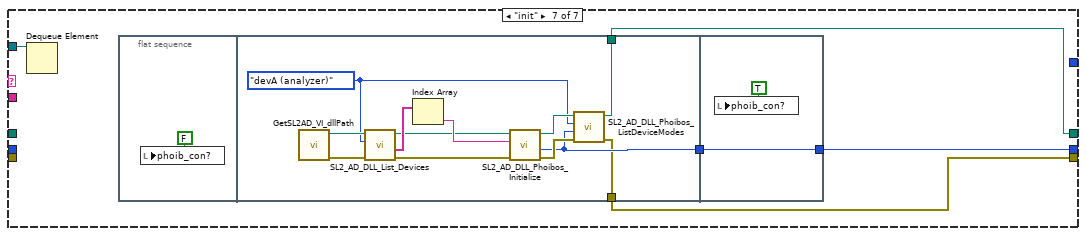
[diagram p17: hidden frame]
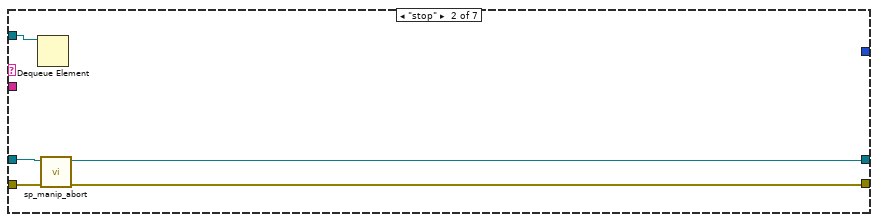
[diagram p18: hidden frame]
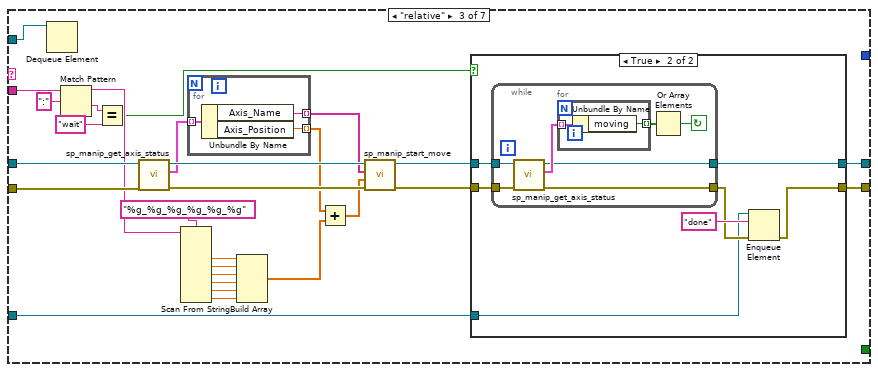
[diagram p19: hidden frame]
diagram:
  w14 = "init" ("name (unnamed)")
  w16 = "" ("name (unnamed)")
  # "scanvector"
  # "imgs"
  # "avg img"
  # "avg"
  # "time"
  # "dark"
  # "Error"
  # "Handle"
  # "memory pointer"
  n1 = Current VI's Path() -> (path=w4:path)
  n2 = Strip Path(path=w4) -> (stripped path=w8:path)  [unwired: 1 out]
  n3 = Strip Path(path=w8) -> (stripped path=w9:path)  [unwired: 1 out]
  n4 = Build Path(base path=w9, name or relative path="runnumber.txt") -> (appended path=w6:path)
  n5 = Obtain Queue(name (unnamed)="dataQ", element data type=dbl[][][] []) -> (queue out=w11:refnum<queue>)  [unwired: 3 in, 2 out]
  n6 = Obtain Queue(name (unnamed)="cam", element data type=w16) -> (queue out=w36:refnum<queue>, error out=w35:errorcluster)  [unwired: 3 in, 1 out]
  n7 = Obtain Queue(name (unnamed)="ESP", element data type=w16) -> (queue out=w33:refnum<queue>, error out=w34:errorcluster)  [unwired: 3 in, 1 out]
  n8 = Obtain Queue(name (unnamed)="manip", element data type=w16) -> (queue out=w30:refnum<queue>, error out=w29:errorcluster)  [unwired: 3 in, 1 out]
  n9 = Obtain Queue(name (unnamed)="phoib", element data type=w16) -> (queue out=w27:refnum<queue>, error out=w28:errorcluster)  [unwired: 3 in, 1 out]
  n10 = Obtain Queue(name (unnamed)="meas", element data type=w16) -> (queue out=w2:refnum<queue>)  [unwired: 3 in, 2 out]
  n11 = Read from Text File(file (use dialog)=w6) -> (text=w7:string)  [unwired: 3 in, 3 out]
  n12 = Enqueue Element(queue=w36, element=w14, error in (no error)=w35) -> (queue out=w10:refnum<queue>)  [unwired: 1 in, 2 out]
  n13 = Enqueue Element(queue=w33, element=w14, error in (no error)=w34) -> (queue out=w13:refnum<queue>)  [unwired: 1 in, 2 out]
  n14 = Enqueue Element(queue=w30, element="suspend" ("name (unnamed)"), error in (no error)=w29) -> (queue out=w3:refnum<queue>)  [unwired: 1 in, 2 out]
  n15 = Enqueue Element(queue=w27, element=w14, error in (no error)=w28) -> (queue out=w24:refnum<queue>)  [unwired: 1 in, 2 out]
  n16 = Decimal String To Number(string=w7) -> (number=w1:i32)  [unwired: 2 in, 1 out]
  n17 = local write "RunNumber"(w1) -> ()
  n18 = while {
    tunnel: w11 -> [w52]
    tunnel: w13 -> [w51]
    tunnel: w10 -> [w50]
    shift-right: [w47] -> _
    shift-left: _ -> [w49]
    shift-right: [w46] -> _
    shift-left: _ -> [w48]
    tunnel: w2 -> [w43]
    tunnel: w3 -> [w38]
    stop <- w39 stop-if-true
    n19 = Preview Queue Element(queue=w43) -> (queue out=w40:refnum<queue>, element=w45:string)  [unwired: 2 in, 2 out]
    n20 = Match Pattern(string=w45, regular expression=":") -> (before substring=w42:string, after substring=w41:string)  [unwired: 1 in, 2 out]
    n21 = case shown="\"GO\"" w42 {
      tunnel: w52 -> [_ _ w86 _ w249 _ w456 w568]
      tunnel: w51 -> [_ _ w85 _ w248 _ _ _]
      tunnel: w50 -> [_ _ w84 _ w247 _ w455 w570]
      tunnel: w49 -> [w54 w58 _ w221 _ w417 w452 w567]
      tunnel: w48 -> [w53 w57 _ w220 _ w415 w451 w566]
      tunnel: [w54 w58 w59 w221 w246 w417 w452 w567] -> w47
      tunnel: [w53 w57 w66 w220 w229 w415 w451 w566] -> w46
      tunnel: w41 -> [_ _ _ _ _ _ _ _]
      tunnel: w40 -> [w56 _ w75 w222 w238 w419 w450 w569]
      tunnel: [TRUE _ _ _ _ _ _ _] -> w39
      tunnel: w38 -> [_ _ _ _ _ _ w454 _]
      frame "close" {
        n22 = Release Queue(queue=w56) -> ()  [unwired: 2 in, 3 out]
      }
      frame "idle", Default {
      }
      frame "GO" {
        n23 = Dequeue Element(queue=w75) -> (queue out=w74:refnum<queue>)  [unwired: 2 in, 3 out]
        n24 = local read "RunNumber"() -> (w81:u16)
        n25 = local read "BasePath"() -> (w80:path)
        n26 = local read "ESP Axis"() -> (w78:i32)
        n27 = local read "ESP_t0"() -> (w64:dbl)
        n28 = Increment(x=w81) -> (x+1=w79:u16)
        n29 = Current VI's Path() -> (path=w82:path)
        n30 = call "2delaypoints.vi"("Offset (mm)"=w64, "delay table [fs]"="delay table [fs]") -> ("delay points [mm]"=w63:dbl[], "delay pointss [fs]"=w61:dbl[])
        n31 = Number To Decimal String(number=w78) -> (decimal integer string=w77:string)  [unwired: 1 in]
        n32 = call "create_opti_path.vi"("RunNumber"=w79, "base path"=w80) -> ("Path"=w71:path)  [unwired: 2 in]
        n33 = call "saverunnumber.vi"("RunNumber"=w79, "VI path"=w82) -> ()  [unwired: 10 in]
        n34 = local write "RunNumber"(w79) -> ()
        n35 = Get Date/Time In Seconds() -> (seconds since 1Jan1904=w60:timestamp)
        n36 = Build Path(base path=w71, name or relative path="info.txt") -> (appended path=w62:path)
        n37 = while {
          tunnel: w63 -> [w123]
          tunnel: w77 -> [w131]
          tunnel: w85 -> [w130]
          tunnel: w86 -> [w129]
          tunnel: w74 -> [w128]
          tunnel: w84 -> [w127]
          tunnel: w71 -> [w126]
          shift-right: [w124] -> w83
          shift-left: dbl[][][] [] -> [w125]
          tunnel: [w122] -> w67
          tunnel: w62 -> [w89]
          tunnel: w61 -> [w88]
          tunnel: w60 -> [w87]
          i -> [w121]
          stop <- w117 stop-if-true
          n38 = for {
            N -> [w153]
            tunnel: w123 -> [w162] mode=indexing
            tunnel: w131 -> [w179]
            tunnel: w130 -> [w178]
            tunnel: w129 -> [w173]
            tunnel: w128 -> [w177]
            tunnel: w127 -> [w176]
            tunnel: w126 -> [w147]
            shift-right: [w137] -> w124
            shift-left: w125 -> [w169]
            tunnel: w121 -> [w146]
            tunnel: w88 -> [w135]
            tunnel: [w135] -> w122
            tunnel: [w159] -> w119
            tunnel: w87 -> [w149]
            tunnel: "delscan_iters" -> [w154]
            i -> [w139]
            stop <- "delscan_abort" stop-if-true
            w181 = ":" ("string")
            # "average data"
            # "init array?"
            n39 = Number To Fractional String(number=w162) -> (F-format string=w171:string)  [unwired: 3 in]
            n40 = property on="delscan_progress" class="Slide (strict)"("Scale.Maximum"=w153) -> ()  [unwired: 2 in, 2 out]
            n41 = Get Date/Time In Seconds() -> (seconds since 1Jan1904=w157:timestamp)
            n42 = call "createFileStruc.vi"("i_iter"=w146, "i_delay"=w139, "meas_path"=w147) -> ("AVG file"=w142:path, "RAW file"=w143:path)  [unwired: 7 in]
            n43 = Concatenate Strings("abs:" ("string"), w179, w181, w171, w181, "wait" ("string")) -> (w184:string)
            n44 = Enqueue Element(queue=w178, element=w184) -> (error out=w182:errorcluster)  [unwired: 2 in, 2 out]
            n45 = Subtract(x=w157, y=w149) -> (x-y=w155:dbl)
            n46 = Equal To 0?(x=w139) -> (x = 0?=w145:bool)
            n47 = Equal To 0?(x=w146) -> (x = 0?=w144:bool)
            n48 = Dequeue Element(queue=w177, error in (no error)=w182) -> (error out=w174:errorcluster)  [unwired: 1 in, 3 out]
            n49 = And(x=w145, y=w144) -> (x .and. y?=w170:bool)
            n50 = Enqueue Element(queue=w176, element="snap", error in (no error)=w174) -> (error out=w172:errorcluster)  [unwired: 1 in, 2 out]
            n51 = Dequeue Element(queue=w173, error in (no error)=w172) -> (element=w165:dbl[][][])  [unwired: 1 in, 3 out]
            n52 = Index Array(array=w165, index (dim 0)=0 ("disabled index (col)")) -> (element=w133:dbl[][])  [unwired: 2 in]
            n53 = Multiply(x=w153, y=w146) -> (x*y=w158:i32)
            n54 = Multiply(x=w153, y=w154) -> (x*y=w152:u32)
            n55 = Array Size(array=w133) -> (size(s)=w166:i32[])
            n56 = Add(x=w158, y=w139) -> (x+y=w156:i32)
            n57 = call-poly <vilib>:"Write Delimited Spreadsheet.vi"("file path (dialog if empty)"=w143, "2D data"=w133) -> ()  [unwired: 12 in, 2 out]
            n58 = Index Array(array=w166) -> (element #1=w164:i32, element #2=w163:i32)  [unwired: 2 in]
            n59 = Divide(x=w155, y=w156) -> (x/y=w151:dbl)
            "time / step" <- w151
            n60 = Multiply(x=w152, y=w151) -> (x*y=w150:dbl)
            n61 = case shown="True" w170 {
              tunnel: w153 -> [_ w193]
              tunnel: [w188 w191] -> w168
              tunnel: w169 -> [w188 _]
              tunnel: w164 -> [_ w190]
              tunnel: w163 -> [_ w189]
              frame False {
              }
              frame True {
                n62 = Initialize Array(0.0 ("element"), w193, w190, w189) -> (w191:dbl[][][])
              }
            }
            n63 = Add(x=w149, y=w150) -> (x+y=→"del_ETA":timestamp)
            n64 = for {
              N: w164 -> [_]
              tunnel: w139 -> [w200]
              shift-right: [w198] -> w137
              shift-left: w168 -> [w201]
              tunnel: w146 -> [w196]
              shift-right: [w195] -> w167
              shift-left: w133 -> [w197]
              tunnel: w163 -> [w194]
              i -> [w199]
              n65 = for {
                N: w194 -> [_]
                tunnel: w200 -> [w208]
                tunnel: w199 -> [w205]
                shift-right: [w207] -> w198
                shift-left: w201 -> [w209]
                tunnel: w196 -> [w203]
                shift-right: [w202] -> w195
                shift-left: w197 -> [w206]
                i -> [w204]
                n66 = in-place {
                  in-place-border: w203 -> [w215]
                  n67 = in-place-array #1(w209, w208, w205, w204) -> (w216:dbl)
                  n68 = in-place-array #2(w206, w205, w204) -> (w213:dbl)
                  n69 = Multiply(x=w216, y=w215) -> (x*y=w214:dbl)
                  n70 = Increment(x=w215) -> (x+1=w211:i32)
                  n71 = Add(x=w214, y=w213) -> (x+y=w212:dbl)
                  n72 = Divide(x=w212, y=w211) -> (x/y=w210:dbl)
                  n73 = in-place-array #1(w210) -> (w207:dbl[][][])  [unwired: 3 out]
                  n74 = in-place-array #2(w210) -> (w202:dbl[][])  [unwired: 2 out]
                }
              }
            }
            n75 = call-poly <vilib>:"Write Delimited Spreadsheet.vi"("file path (dialog if empty)"=w142, "2D data"=w167) -> ()  [unwired: 12 in, 2 out]
            n76 = property on="mainimg" class="IntGraph (strict)"() -> ("CrsrLis"=w138:T5)  [unwired: 2 in, 2 out]
            n77 = call "processData.vi"("Cursor List"=w138, "data in"=w137) -> ("Intensity Chart"=w136:dbl[])  [unwired: 1 in, 2 out]
            n78 = Increment(x=w139) -> (x+1=w140:i32)
            n79 = Bundle("delay pointss [fs]"=w135, "Intensity Chart"=w136) -> (w134:T6)  [unwired: 1 in]
            n80 = flat-sequence {
              tunnel: w134 -> [w186]
              tunnel: [w185] -> w141
              tunnel: w140 -> [w187]
              frame #0 {
                n81 = Build Array(w186) -> (w185:T3)
                "delscan_progress" <- w187
              }
            }
            n82 = Or(x="delscan_finishIteration", y="delscan_abort") -> (x .or. y?=w159:bool)
            "delscan_pos" <- w162
            "scangraph" <- w141
          }
          n83 = Increment(x=w121) -> (x+1=w120:i32)
          "iteration" <- w120
          n84 = local read "exposure [ms]"() -> (w104:u32)
          n85 = local read "ROI Bottom"() -> (w107:i32)
          n86 = local read "iteration"() -> (w114:i32)
          n87 = property on="Mode" class="Enum (strict)"() -> ("RingText.Text"=w93:string)  [unwired: 2 in, 2 out]
          n88 = property on="VoltageRange" class="Enum (strict)"() -> ("RingText.Text"=w94:string)  [unwired: 2 in, 2 out]
          n89 = local read "cam_dark?"() -> (w91:bool)
          n90 = local read "phoib_I_1"() -> (w95:dbl)
          n91 = local read "phoib_I_2"() -> (w96:dbl)
          n92 = local read "phoib_I_3"() -> (w97:dbl)
          n93 = local read "phoib_I_4"() -> (w98:dbl)
          n94 = local read "phoib_I_5"() -> (w99:dbl)
          n95 = local read "phoib_I_6"() -> (w100:dbl)
          n96 = local read "phoib_I_7"() -> (w101:dbl)
          n97 = local read "phoib_I_8"() -> (w102:dbl)
          n98 = local read "phoib_I_9"() -> (w103:dbl)
          n99 = local read "ROI Right"() -> (w109:i32)
          n100 = local read "averages"() -> (w113:i32)
          n101 = local read "ROI Top"() -> (w108:i32)
          n102 = local read "ROI Left"() -> (w110:i32)
          n103 = local read "binning"() -> (w106:u16)
          n104 = local read "ESP_t0"() -> (w115:dbl)
          n105 = local read "gain"() -> (w90:bool)
          n106 = Boolean To (0,1)(Boolean=w90) -> (0, 1=w105:i16)
          n107 = Boolean To (0,1)(Boolean=w91) -> (0, 1=w111:i16)
          n108 = Format Into String(format string="ScanType:%s\\nAverages:%u\\nRepetitions:%u\\nTimeZero:%f\\nLensMode:%s\\nVoltageRange:%s\\nKineticEnergy:%f\\nPassEnergy:%f\\nCoilCurrent:%f\\nWorkFunction:%f\\nDetectorVoltage:%f\\nScreenVoltage:%f\\nConversionVoltage:%f\\nFocusDisplacement1:%f\\nFocusDisplacement2:%f\\nExposure:%u\\nGain:%u\\nBinning:%u\\nROIbottom:%u\\nROItop:%u\\nROIright:%u\\nROIleft:%u\\nDarkImg:%u\\nStartTime:%<%Y.%m.%d %H:%M:%S>T", initial string=w89, "delay" ("input 1"), w113, w114, w115, w93, w94, w95, w96, w97, w98, w99, w100, w101, w102, w103, w104, w105, w106, w107, w108, w109, w110, w111, w87) -> ()  [unwired: 1 in, 2 out]
          n109 = Less Or Equal?(x="delscan_iters", y=w120) -> (x <= y?=w118:bool)
          n110 = Or(x=w119, y=w118) -> (x .or. y?=w117:bool)
        }
        n111 = Build Path(base path=w71, name or relative path="scanvector.txt") -> (appended path=w68:path)
        n112 = call-poly <vilib>:"Write Delimited Spreadsheet.vi"("file path (dialog if empty)"=w68, "format (%.3f)"="%.6f", "1D data"=w63, "transpose? (F)"=TRUE) -> ()  [unwired: 10 in, 2 out]
        n113 = flat-sequence {
          tunnel: w67 -> [w219]
          tunnel: [w219] -> w66
          frame #0 {
            w218 = u32 1000 ("frequency (Hz)")
            n114 = call <vilib>:"Beep.vi"("use system alert? (T)"=FALSE, "duration (msec)"=w218, "frequency (Hz)"=w218) -> ()  [unwired: 9 in]
          }
        }
        n115 = Build Array(w83) -> (w59:dbl[][][][])
      }
      frame "done" {
        n116 = Dequeue Element(queue=w222) -> ()  [unwired: 2 in, 4 out]
      }
      frame "delay_chop" {
        n117 = local read "delay table [fs]"() -> (w223:string[][])
        n118 = Dequeue Element(queue=w238) -> (queue out=w237:refnum<queue>)  [unwired: 2 in, 3 out]
        n119 = local read "RunNumber"() -> (w244:u16)
        n120 = local read "BasePath"() -> (w243:path)
        n121 = local read "ESP Axis"() -> (w241:i32)
        n122 = local read "ESP_t0"() -> (w228:dbl)
        n123 = Increment(x=w244) -> (x+1=w242:u16)
        n124 = Current VI's Path() -> (path=w245:path)
        n125 = call "2delaypoints.vi"("Offset (mm)"=w228, "delay table [fs]"=w223) -> ("delay points [mm]"=w227:dbl[], "delay pointss [fs]"=w225:dbl[])
        n126 = Number To Decimal String(number=w241) -> (decimal integer string=w240:string)  [unwired: 1 in]
        n127 = call "create_opti_path.vi"("RunNumber"=w242, "base path"=w243) -> ("Path"=w234:path)  [unwired: 2 in]
        n128 = call "saverunnumber.vi"("RunNumber"=w242, "VI path"=w245) -> ()  [unwired: 10 in]
        n129 = local write "RunNumber"(w242) -> ()
        n130 = Get Date/Time In Seconds() -> (seconds since 1Jan1904=w224:timestamp)
        n131 = Build Path(base path=w234, name or relative path="info.txt") -> (appended path=w226:path)
        n132 = while {
          tunnel: w227 -> [w286]
          tunnel: w240 -> [w294]
          tunnel: w248 -> [w293]
          tunnel: w249 -> [w292]
          tunnel: w237 -> [w291]
          tunnel: w247 -> [w290]
          tunnel: w234 -> [w289]
          shift-right: [w287] -> w246
          shift-left: dbl[][][][] [] -> [w288]
          tunnel: [w285] -> w230
          tunnel: w226 -> [w254]
          tunnel: w225 -> [w253]
          tunnel: w224 -> [w252]
          i -> [w284]
          stop <- w281 stop-if-true
          n133 = Increment(x=w284) -> (x+1=w251:i32)
          n134 = local read "exposure [ms]"() -> (w269:u32)
          n135 = local read "ROI Bottom"() -> (w272:i32)
          n136 = local read "iteration"() -> (w279:i32)
          n137 = property on="Mode" class="Enum (strict)"() -> ("RingText.Text"=w258:string)  [unwired: 2 in, 2 out]
          n138 = property on="VoltageRange" class="Enum (strict)"() -> ("RingText.Text"=w259:string)  [unwired: 2 in, 2 out]
          n139 = local read "cam_dark?"() -> (w256:bool)
          n140 = local write "iteration"(w251) -> ()
          n141 = local read "phoib_I_1"() -> (w260:dbl)
          n142 = local read "phoib_I_2"() -> (w261:dbl)
          n143 = local read "phoib_I_3"() -> (w262:dbl)
          n144 = local read "phoib_I_4"() -> (w263:dbl)
          n145 = local read "phoib_I_5"() -> (w264:dbl)
          n146 = local read "phoib_I_6"() -> (w265:dbl)
          n147 = local read "phoib_I_7"() -> (w266:dbl)
          n148 = local read "phoib_I_8"() -> (w267:dbl)
          n149 = local read "phoib_I_9"() -> (w268:dbl)
          n150 = local read "ROI Right"() -> (w274:i32)
          n151 = local read "averages"() -> (w278:i32)
          n152 = local read "ROI Top"() -> (w273:i32)
          n153 = local read "ROI Left"() -> (w275:i32)
          n154 = local read "binning"() -> (w271:u16)
          n155 = local read "ESP_t0"() -> (w280:dbl)
          n156 = local read "gain"() -> (w255:bool)
          n157 = Boolean To (0,1)(Boolean=w255) -> (0, 1=w270:i16)
          n158 = Boolean To (0,1)(Boolean=w256) -> (0, 1=w276:i16)
          n159 = local read "delscan_iters"() -> (w250:u32)
          n160 = for {
            N -> [w328]
            tunnel: w286 -> [w325] mode=indexing
            tunnel: w294 -> [w357]
            tunnel: w293 -> [w356]
            tunnel: w292 -> [w351]
            tunnel: w291 -> [w355]
            tunnel: w290 -> [w354]
            tunnel: w289 -> [w335]
            shift-right: [w315] -> w287
            shift-left: w288 -> [w347]
            tunnel: w284 -> [w334]
            tunnel: w253 -> [w312]
            tunnel: [w312] -> w285
            tunnel: [w344] -> w283
            tunnel: w252 -> [w336]
            tunnel: w250 -> [w339]
            i -> [w330]
            stop <- "delscan_abort 2" stop-if-true
            w359 = ":" ("string")
            # "init array?"
            n161 = local write "delscan_pos"(w325) -> ()
            n162 = Number To Fractional String(number=w325) -> (F-format string=w349:string)  [unwired: 3 in]
            n163 = Get Date/Time In Seconds() -> (seconds since 1Jan1904=w342:timestamp)
            n164 = call "createFileStrucChop.vi"("i_iter"=w334, "i_delay"=w330, "meas_path"=w335) -> ("AVG file off"=w295:path, "AVG file on"=w296:path, "RAW file off"=w297:path, "RAW file on"=w298:path)  [unwired: 3 in]
            n165 = property on="delscan_progress" class="Slide (strict)"("Scale.Maximum"=w328) -> ()  [unwired: 2 in, 2 out]
            n166 = Concatenate Strings("abs:" ("string"), w357, w359, w349, w359, "wait" ("string")) -> (w362:string)
            n167 = Enqueue Element(queue=w356, element=w362) -> (error out=w360:errorcluster)  [unwired: 2 in, 2 out]
            n168 = Subtract(x=w342, y=w336) -> (x-y=w340:dbl)
            n169 = Equal To 0?(x=w330) -> (x = 0?=w333:bool)
            n170 = Equal To 0?(x=w334) -> (x = 0?=w332:bool)
            n171 = Dequeue Element(queue=w355, error in (no error)=w360) -> (error out=w352:errorcluster)  [unwired: 1 in, 3 out]
            n172 = And(x=w333, y=w332) -> (x .and. y?=w348:bool)
            n173 = Enqueue Element(queue=w354, element="snap", error in (no error)=w352) -> (error out=w350:errorcluster)  [unwired: 1 in, 2 out]
            n174 = Dequeue Element(queue=w351, error in (no error)=w350) -> (element=w320:dbl[][][])  [unwired: 1 in, 3 out]
            n175 = Multiply(x=w328, y=w334) -> (x*y=w343:i32)
            n176 = Multiply(x=w328, y=w339) -> (x*y=w338:u32)
            n177 = Index Array(array=w320, index (dim 0)=1 ("disabled index (col)")) -> (element=w322:dbl[][])  [unwired: 2 in]
            n178 = Array Size(array=w320) -> (size(s)=w345:i32[])
            n179 = Index Array(array=w320, index (dim 0)=0 ("disabled index (col)")) -> (element=w321:dbl[][])  [unwired: 2 in]
            n180 = Add(x=w343, y=w330) -> (x+y=w341:i32)
            n181 = Index Array(array=w345) -> (element #1=w301:i32, element #2=w300:i32, element #3=w299:i32)  [unwired: 3 in]
            n182 = Divide(x=w340, y=w341) -> (x/y=w326:dbl)
            n183 = call-poly <vilib>:"Write Delimited Spreadsheet.vi"("file path (dialog if empty)"=w297, "2D data"=w322) -> ()  [unwired: 12 in, 2 out]
            n184 = call-poly <vilib>:"Write Delimited Spreadsheet.vi"("file path (dialog if empty)"=w298, "2D data"=w321) -> ()  [unwired: 12 in, 2 out]
            n185 = Multiply(x=w338, y=w326) -> (x*y=w337:dbl)
            n186 = case shown="True" w348 {
              tunnel: w328 -> [_ w407]
              tunnel: [w401 w405] -> w346
              tunnel: w347 -> [w401 _]
              tunnel: w301 -> [_ w404]
              tunnel: w300 -> [_ w403]
              tunnel: w299 -> [_ w402]
              frame False {
              }
              frame True {
                n187 = Initialize Array(0.0 ("element"), w407, w404, w403, w402) -> (w405:dbl[][][][])
              }
            }
            n188 = Add(x=w336, y=w337) -> (x+y=w327:timestamp)
            n189 = local write "del_ETA"(w327) -> ()
            n190 = local write "time / step"(w326) -> ()
            n191 = for {
              N: w301 -> [_]
              tunnel: w300 -> [w368]
              tunnel: w299 -> [w367]
              tunnel: w334 -> [w366]
              tunnel: w330 -> [w365]
              shift-right: [w364] -> w315
              shift-left: w346 -> [w371]
              shift-right: [w370] -> w318
              shift-left: w320 -> [w369]
              i -> [w363]
              # "average data"
              n192 = for {
                N: w368 -> [_]
                tunnel: w365 -> [w379]
                shift-right: [w377] -> w364
                shift-left: w371 -> [w380]
                tunnel: w366 -> [w375]
                shift-right: [w374] -> w370
                shift-left: w369 -> [w376]
                tunnel: w367 -> [w373]
                tunnel: w363 -> [w372]
                i -> [w378]
                n193 = for {
                  N: w373 -> [_]
                  tunnel: w379 -> [w382]
                  tunnel: w378 -> [w383]
                  shift-right: [w388] -> w377
                  shift-left: w380 -> [w389]
                  tunnel: w375 -> [w386]
                  shift-right: [w385] -> w374
                  shift-left: w376 -> [w387]
                  tunnel: w372 -> [w381]
                  i -> [w384]
                  n194 = in-place {
                    in-place-border: w386 -> [w395]
                    n195 = in-place-array #3(w389, w382, w381, w383, w384) -> (w396:dbl)
                    n196 = in-place-array #4(w387, w381, w383, w384) -> (w393:dbl)
                    n197 = Multiply(x=w396, y=w395) -> (x*y=w394:dbl)
                    n198 = Increment(x=w395) -> (x+1=w391:i32)
                    n199 = Add(x=w394, y=w393) -> (x+y=w392:dbl)
                    n200 = Divide(x=w392, y=w391) -> (x/y=w390:dbl)
                    n201 = in-place-array #3(w390) -> (w388:dbl[][][][])  [unwired: 4 out]
                    n202 = in-place-array #4(w390) -> (w385:dbl[][][])  [unwired: 3 out]
                  }
                }
              }
            }
            n203 = Index Array(array=w318, index (dim 0)=0 ("disabled index (col)")) -> (element=w319:dbl[][])  [unwired: 2 in]
            n204 = Index Array(array=w318, index (dim 0)=1 ("disabled index (col)")) -> (element=w317:dbl[][])  [unwired: 2 in]
            n205 = call-poly <vilib>:"Write Delimited Spreadsheet.vi"("file path (dialog if empty)"=w296, "2D data"=w319) -> ()  [unwired: 12 in, 2 out]
            n206 = call-poly <vilib>:"Write Delimited Spreadsheet.vi"("file path (dialog if empty)"=w295, "2D data"=w317) -> ()  [unwired: 12 in, 2 out]
            n207 = Index Array(array=w315, index (dim 1)=1 ("disabled index (col)")) -> (element=w314:dbl[][][])  [unwired: 3 in]
            n208 = Index Array(array=w315, index (dim 1)=0 ("disabled index (col)")) -> (element=w316:dbl[][][])  [unwired: 3 in]
            n209 = Increment(x=w330) -> (x+1=w331:i32)
            n210 = property on="mainimg" class="IntGraph (strict)"() -> ("CrsrLis"=w313:T5)  [unwired: 2 in, 2 out]
            n211 = call "processData.vi"("Cursor List"=w313, "data in"=w316) -> ("Intensity Chart"=w329:dbl[])  [unwired: 1 in, 2 out]
            n212 = call "processData.vi"("Cursor List"=w313, "data in"=w314) -> ("Intensity Chart"=w311:dbl[])  [unwired: 1 in, 2 out]
            n213 = Bundle("delay pointss [fs]"=w312, "Intensity Chart"=w329) -> (w310:T6)  [unwired: 1 in]
            n214 = Bundle("delay pointss [fs]"=w312, "Intensity Chart"=w311) -> (w309:T6)  [unwired: 1 in]
            n215 = flat-sequence {
              tunnel: w331 -> [w400]
              tunnel: w310 -> [w399]
              tunnel: w309 -> [w397]
              tunnel: [w398] -> w302
              frame #0 {
                n216 = local write "delscan_progress"(w400) -> ()
                n217 = Build Array(w399, w397) -> (w398:T3)
              }
            }
            n218 = Or(x="delscan_finishIteration 2", y="delscan_abort 2") -> (x .or. y?=w344:bool)
            n219 = local write "scangraph"(w302) -> ()
          }
          n220 = Format Into String(format string="ScanType:%s\\nAverages:%u\\nRepetitions:%u\\nTimeZero:%f\\nLensMode:%s\\nVoltageRange:%s\\nKineticEnergy:%f\\nPassEnergy:%f\\nCoilCurrent:%f\\nWorkFunction:%f\\nDetectorVoltage:%f\\nScreenVoltage:%f\\nConversionVoltage:%f\\nFocusDisplacement1:%f\\nFocusDisplacement2:%f\\nExposure:%u\\nGain:%u\\nBinning:%u\\nROIbottom:%u\\nROItop:%u\\nROIright:%u\\nROIleft:%u\\nDarkImg:%u\\nStartTime:%<%Y.%m.%d %H:%M:%S>T", initial string=w254, "delay_chop" ("input 1"), w278, w279, w280, w258, w259, w260, w261, w262, w263, w264, w265, w266, w267, w268, w269, w270, w271, w272, w273, w274, w275, w276, w252) -> ()  [unwired: 1 in, 2 out]
          n221 = Less Or Equal?(x=w250, y=w251) -> (x <= y?=w282:bool)
          n222 = Or(x=w283, y=w282) -> (x .or. y?=w281:bool)
        }
        n223 = Build Path(base path=w234, name or relative path="scanvector.txt") -> (appended path=w231:path)
        n224 = call-poly <vilib>:"Write Delimited Spreadsheet.vi"("file path (dialog if empty)"=w231, "format (%.3f)"="%.6f", "1D data"=w227, "transpose? (F)"=TRUE) -> ()  [unwired: 10 in, 2 out]
        n225 = flat-sequence {
          tunnel: w230 -> [w410]
          tunnel: [w410] -> w229
          frame #0 {
            w409 = u32 1000 ("frequency (Hz)")
            n226 = call <vilib>:"Beep.vi"("use system alert? (T)"=FALSE, "duration (msec)"=w409, "frequency (Hz)"=w409) -> ()  [unwired: 9 in]
          }
        }
      }
      frame "refresh" {
        n227 = Dequeue Element(queue=w419) -> ()  [unwired: 2 in, 4 out]
        n228 = property on="mainimg" class="IntGraph (strict)"() -> ("CrsrLis"=w418:T5)  [unwired: 2 in, 2 out]
        n229 = Index Array(array=w417, index (dim 0)=0 ("disabled index (col)")) -> (element=w414:dbl[][][])  [unwired: 3 in]
        n230 = call "processData.vi"("Cursor List"=w418, "data in"=w414) -> ("Intensity Chart"=w416:dbl[])  [unwired: 1 in, 2 out]
        n231 = Bundle("delay pointss [fs]"=w415, "Intensity Chart"=w416) -> (w413:T6)  [unwired: 1 in]
        n232 = Build Array(w413) -> (w412:T3)
        n233 = local write "scangraph"(w412) -> ()
      }
      frame "manip" {
        n234 = Dequeue Element(queue=w450) -> (queue out=w449:refnum<queue>)  [unwired: 2 in, 3 out]
        n235 = local read "RunNumber"() -> (w458:u16)
        n236 = local read "BasePath"() -> (w459:path)
        n237 = property on="delscan_progress 2" class="Slide (strict)"("Scale.Maximum"="manip_scan_steps") -> ()  [unwired: 2 in, 2 out]
        n238 = Index Array(array="manip_scan_delta") -> (element #1=w471:dbl, element #2=w470:dbl, element #3=w469:dbl, element #4=w468:dbl, element #5=w467:dbl, element #6=w466:dbl)  [unwired: 6 in]
        n239 = Increment(x=w458) -> (x+1=w460:u16)
        n240 = Current VI's Path() -> (path=w457:path)
        n241 = Format Into String(format string="%g_%g_%g_%g_%g_%g", w471, w470, w469, w468, w467, w466) -> (resulting string=w464:string)  [unwired: 2 in, 1 out]
        n242 = property on="Mode" class="Enum (strict)"() -> ("RingText.Text"=w444:string)  [unwired: 2 in, 2 out]
        n243 = property on="VoltageRange" class="Enum (strict)"() -> ("RingText.Text"=w443:string)  [unwired: 2 in, 2 out]
        n244 = call "saverunnumber.vi"("RunNumber"=w460, "VI path"=w457) -> ()  [unwired: 10 in]
        n245 = local write "RunNumber"(w460) -> ()
        n246 = call "create_opti_path.vi"("RunNumber"=w460, "base path"=w459) -> ("Path"=w423:path)  [unwired: 2 in]
        n247 = local read "exposure [ms]"() -> (w433:u32)
        n248 = Build Path(base path=w423, name or relative path="info.txt") -> (appended path=w422:path)
        n249 = Concatenate Strings("relative:" ("string"), w464, ":wait" ("string")) -> (w473:string)
        n250 = local read "ROI Bottom"() -> (w430:i32)
        n251 = local read "cam_dark?"() -> (w447:bool)
        n252 = local read "phoib_I_1"() -> (w442:dbl)
        n253 = local read "phoib_I_2"() -> (w441:dbl)
        n254 = local read "phoib_I_3"() -> (w440:dbl)
        n255 = local read "phoib_I_4"() -> (w439:dbl)
        n256 = local read "phoib_I_5"() -> (w438:dbl)
        n257 = local read "phoib_I_6"() -> (w437:dbl)
        n258 = local read "phoib_I_7"() -> (w436:dbl)
        n259 = local read "phoib_I_8"() -> (w435:dbl)
        n260 = local read "phoib_I_9"() -> (w434:dbl)
        n261 = local read "ROI Right"() -> (w428:i32)
        n262 = local read "averages"() -> (w445:i32)
        n263 = local read "ROI Top"() -> (w429:i32)
        n264 = local read "ROI Left"() -> (w427:i32)
        n265 = local read "binning"() -> (w431:u16)
        n266 = local read "gain"() -> (w448:bool)
        n267 = Get Date/Time In Seconds() -> (seconds since 1Jan1904=w425:timestamp)
        n268 = Build Path(base path=w423, name or relative path="scanvector.txt") -> (appended path=w474:path)
        n269 = for {
          N: 1 -> [_]
          tunnel: w456 -> [w489]
          tunnel: w423 -> [w488]
          tunnel: w474 -> [w481]
          tunnel: "manip_scan_steps" -> [w480]
          tunnel: w473 -> [w479]
          tunnel: w454 -> [w478]
          tunnel: w449 -> [w477]
          tunnel: w455 -> [w476]
          tunnel: "manip_scan_delta" -> [w475]
          i -> [w483]
          n270 = Add(x=w483, y=1000) -> (x+y=w486:i32)
          n271 = Number To Decimal String(number=w486) -> (decimal integer string=w485:string)  [unwired: 1 in]
          n272 = String Subset(string=w485, offset (0)=1) -> (substring=w482:string)  [unwired: 1 in]
          n273 = for {
            N: w480 -> [_]
            tunnel: w489 -> [w514]
            tunnel: w488 -> [w511]
            tunnel: w482 -> [w505]
            tunnel: w481 -> [w507]
            tunnel: w479 -> [w502]
            tunnel: w478 -> [w501]
            tunnel: w477 -> [w500]
            tunnel: w476 -> [w499]
            tunnel: w475 -> [w497]
            i -> [w492]
            stop <- "abort" stop-if-true
            n274 = Increment(x=w492) -> (x+1=→"delscan_progress 2":i32)
            n275 = Multiply(x=w497, y=w492) -> (x*y=w496:dbl[])
            n276 = Enqueue Element(queue=w501, element=w502) -> (error out=w503:errorcluster)  [unwired: 2 in, 2 out]
            n277 = Add(x=w492, y=10000) -> (x+y=w520:i32)
            n278 = Dequeue Element(queue=w500, error in (no error)=w503) -> (error out=w498:errorcluster)  [unwired: 1 in, 3 out]
            n279 = Number To Decimal String(number=w520) -> (decimal integer string=w519:string)  [unwired: 1 in]
            n280 = String Subset(string=w519, offset (0)=1) -> (substring=w504:string)  [unwired: 1 in]
            n281 = Enqueue Element(queue=w499, element="snap", error in (no error)=w498) -> (error out=w513:errorcluster)  [unwired: 1 in, 2 out]
            n282 = Concatenate Strings("RAW\\" ("string"), w505, "_" ("string"), w504, ".tsv" ("string")) -> (w510:string)
            n283 = Dequeue Element(queue=w514, error in (no error)=w513) -> (element=w509:dbl[][][])  [unwired: 1 in, 3 out]
            n284 = Build Path(base path=w511, name or relative path=w510) -> (appended path=w512:path)
            n285 = Index Array(array=w509, index (dim 2)=0 ("disabled index (col)")) -> (element=w491:dbl[][])  [unwired: 2 in]
            n286 = call-poly <vilib>:"Write Delimited Spreadsheet.vi"("file path (dialog if empty)"=w512, "2D data"=w491) -> ()  [unwired: 12 in, 2 out]
            n287 = call-poly <vilib>:"Write Delimited Spreadsheet.vi"("file path (dialog if empty)"=w507, "1D data"=w496, "append to file? (F)"=TRUE, "transpose? (F)"=FALSE) -> ()  [unwired: 10 in, 2 out]
          }
        }
        n288 = Boolean To (0,1)(Boolean=w448) -> (0, 1=w432:i16)
        n289 = Boolean To (0,1)(Boolean=w447) -> (0, 1=w426:i16)
        n290 = Format Into String(format string="ScanType:%s\\nAverages:%u\\nMode:%s\\nVoltageRange:%s\\nKineticEnergy:%f\\nPassEnergy:%f\\nCoilCurrent:%f\\nWorkFunction:%f\\nDetectorVoltage:%f\\nScreenVoltage:%f\\nConversionVoltage:%f\\nFocusDisplacement1:%f\\nFocusDisplacement2:%f\\nExposure:%u\\nGain:%u\\nBinning:%u\\nROIbottom:%u\\nROItop:%u\\nROIright:%u\\nROIleft:%u\\nDarkImg:%u\\nStartTime:%<%Y.%m.%d %H:%M:%S>T", initial string=w422, "manipulator" ("input 1"), w445, w444, w443, w442, w441, w440, w439, w438, w437, w436, w435, w434, w433, w432, w431, w430, w429, w428, w427, w426, w425) -> ()  [unwired: 1 in, 2 out]
      }
      frame "single" {
        n291 = Dequeue Element(queue=w569) -> ()  [unwired: 2 in, 4 out]
        n292 = property on="Mode" class="Enum (strict)"() -> ("RingText.Text"=w555:string)  [unwired: 2 in, 2 out]
        n293 = property on="VoltageRange" class="Enum (strict)"() -> ("RingText.Text"=w554:string)  [unwired: 2 in, 2 out]
        n294 = local read "RunNumber"() -> (w561:u16)
        n295 = local read "BasePath"() -> (w562:path)
        n296 = local read "exposure [ms]"() -> (w544:u32)
        n297 = local read "ROI Bottom"() -> (w541:i32)
        n298 = local read "cam_dark?"() -> (w558:bool)
        n299 = local read "phoib_I_1"() -> (w553:dbl)
        n300 = local read "phoib_I_2"() -> (w552:dbl)
        n301 = local read "phoib_I_3"() -> (w551:dbl)
        n302 = local read "phoib_I_4"() -> (w550:dbl)
        n303 = local read "phoib_I_5"() -> (w549:dbl)
        n304 = local read "phoib_I_6"() -> (w548:dbl)
        n305 = local read "phoib_I_7"() -> (w547:dbl)
        n306 = local read "phoib_I_8"() -> (w546:dbl)
        n307 = local read "phoib_I_9"() -> (w545:dbl)
        n308 = local read "ROI Right"() -> (w539:i32)
        n309 = local read "ESP_pos"() -> (w529:dbl)
        n310 = local read "averages"() -> (w556:i32)
        n311 = local read "ROI Top"() -> (w540:i32)
        n312 = local read "ROI Left"() -> (w538:i32)
        n313 = local read "binning"() -> (w542:u16)
        n314 = local read "ESP_t0"() -> (w530:dbl)
        n315 = Increment(x=w561) -> (x+1=w563:u16)
        n316 = Current VI's Path() -> (path=w560:path)
        n317 = local read "gain"() -> (w559:bool)
        n318 = Get Date/Time In Seconds() -> (seconds since 1Jan1904=w536:timestamp)
        n319 = call "saverunnumber.vi"("RunNumber"=w563, "VI path"=w560) -> ()  [unwired: 10 in]
        n320 = local write "RunNumber"(w563) -> ()
        n321 = call "create_opti_path.vi"("RunNumber"=w563, "base path"=w562) -> ("Path"=w527:path)  [unwired: 2 in]
        n322 = Boolean To (0,1)(Boolean=w559) -> (0, 1=w543:i16)
        n323 = Boolean To (0,1)(Boolean=w558) -> (0, 1=w537:i16)
        n324 = Build Path(base path=w527, name or relative path="info.txt") -> (appended path=w532:path)
        n325 = Format Into String(format string="ScanType=%s\\nDelayPosition=%.6f\\nTimeZero=%.6f\\nAverages=%u\\nLensMode=%s\\nVoltageRange=%s\\nKineticEnergy=%f\\nPassEnergy=%f\\nCoilCurrent=%f\\nWorkFunction=%f\\nDetectorVoltage=%f\\nScreenVoltage=%f\\nConversionVoltage=%f\\nFocusDisplacement1=%f\\nFocusDisplacement2=%f\\nExposure=%u\\nGain=%u\\nBinning=%u\\nROIbottom=%u\\nROItop=%u\\nROIright=%u\\nROIleft=%u\\nDarkImg=%u\\nStartTime=%<%Y.%m.%d %H:%M:%S>T", initial string=w532, "single" ("input 1"), w529, w530, w556, w555, w554, w553, w552, w551, w550, w549, w548, w547, w546, w545, w544, w543, w542, w541, w540, w539, w538, w537, w536) -> ()  [unwired: 1 in, 2 out]
        n326 = local read "Enable Chopping"() -> (w522:bool)
        n327 = Build Path(base path=w527, name or relative path="AVG\\000.tsv") -> (appended path=w534:path)
        n328 = Build Path(base path=w527, name or relative path="AVG\\000_nl.tsv") -> (appended path=w524:path)
        n329 = Enqueue Element(queue=w570, element="snap" ("string")) -> (error out=w564:errorcluster)  [unwired: 2 in, 2 out]
        n330 = Dequeue Element(queue=w568, error in (no error)=w564) -> (element=w526:dbl[][][])  [unwired: 1 in, 3 out]
        n331 = case shown="True" w522 {
          tunnel: w526 -> [_ w573]
          tunnel: w524 -> [_ w571]
          frame False {
          }
          frame True {
            n332 = Index Array(array=w573, index (dim 0)=1 ("disabled index (col)")) -> (element=w574:dbl[][])  [unwired: 2 in]
            n333 = call-poly <vilib>:"Write Delimited Spreadsheet.vi"("file path (dialog if empty)"=w571, "2D data"=w574) -> ()  [unwired: 12 in, 2 out]
          }
        }
        n334 = Index Array(array=w526, index (dim 0)=0 ("disabled index (col)")) -> (element=w528:dbl[][])  [unwired: 2 in]
        n335 = call-poly <vilib>:"Write Delimited Spreadsheet.vi"("file path (dialog if empty)"=w534, "2D data"=w528) -> ()  [unwired: 12 in, 2 out]
      }
    }
  }
  n336 = while {
    tunnel: w10 -> [w601]
    shift-right: [w595] -> _
    shift-left: _ -> [w594]
    shift-right: [w593] -> _
    shift-left: _ -> [w591]
    shift-right: [w592] -> _
    shift-left: _ -> [w590]
    shift-right: [w587] -> _
    shift-left: 0 -> [w588]
    shift-right: [w586] -> _
    shift-left: _ -> [w585]
    shift-right: [w584] -> _
    shift-left: _ -> [w583]
    tunnel: w11 -> [w582]
    shift-right: [w581] -> _
    shift-left: _ -> [w580]
    shift-right: [w578] -> _
    shift-left: _ -> [w577]
    shift-right: [w576] -> _
    shift-left: _ -> [w575]
    i -> [w579]
    stop <- w589 stop-if-true
    # "cam"
    n337 = Preview Queue Element(queue=w601, timeout in ms (-1)=w588) -> (queue out=w600:refnum<queue>, element=w599:string)  [unwired: 1 in, 2 out]
    n338 = Match Pattern(string=w599, regular expression=":") -> (before substring=w596:string, after substring=w597:string)  [unwired: 1 in, 2 out]
    n339 = case shown="\"bench\"" w596 {
      tunnel: w600 -> [w613 w645 w675 w715 w728 _ w816 w849 w991]
      tunnel: w597 -> [_ _ _ _ _ _ _ _ _]
      tunnel: [w607 w632 w671 w714 w726 w769 w813 w834 w989] -> w595
      tunnel: w594 -> [_ _ w671 w714 w726 w769 w813 w834 w989]
      tunnel: [w612 w646 w681 u64 0 ("Hout") w725 w773 w814 w844 w988] -> w593
      tunnel: [w614 w647 w682 w711 w724 w774 w815 w835 w987] -> w592
      tunnel: w591 -> [_ w649 w685 w713 w725 w776 w818 w846 w988]
      tunnel: w590 -> [_ w648 w677 _ w724 w775 w817 w845 w987]
      tunnel: [_ _ _ _ TRUE _ _ _ _] -> w589
      tunnel: [_ _ _ _ _ _ _ _ -1] -> w587
      tunnel: [w606 w633 w676 _ _ w783 _ _ _] -> w586
      tunnel: w585 -> [w606 w633 w676 _ _ w782 _ _ _]
      tunnel: [w607 w635 w678 w709 w723 w778 w807 w847 w986] -> w584
      tunnel: w583 -> [_ w635 w678 w709 w723 w778 _ w847 w986]
      tunnel: w582 -> [_ _ _ _ _ _ _ w838 _]
      tunnel: [w604 w630 w680 w708 w721 w736 w804 w841 w985] -> w581
      tunnel: w580 -> [w604 w630 w680 w708 w721 w771 w804 w841 w985]
      tunnel: w579 -> [_ _ _ _ _ w744 _ _ _]
      tunnel: [w605 w631 w679 w707 w722 w770 w803 w840 w984] -> w578
      tunnel: w577 -> [w605 w631 w679 w707 w722 w743 w803 w840 w984]
      tunnel: [w603 w627 w665 refnum<k21> refnum ("task out") w720 w729 w802 w831 w983] -> w576
      tunnel: w575 -> [_ w627 w666 w706 w720 w729 w802 w832 w983]
      frame "init" {
        w607 = u16[][] []
        n340 = flat-sequence {
          tunnel: [w616] -> w611
          tunnel: [w617] -> w610
          tunnel: [w625] -> w612
          tunnel: [w626] -> w614
          tunnel: w611 -> [w626]
          tunnel: w610 -> [w625]
          frame #0 {
            n341 = local write "cam_con?"(FALSE ("cam_con?")) -> ()
          }
          frame #1 {
            n342 = call "SCInitBoard.vi"("boardnr"="board number") -> ("Hout"=w620:u32, "error out"=w621:errorcluster)  [unwired: 1 in, 1 out]
            n343 = call "SCSetupCamera.vi"("Handle"=w620, "error in (no error)"=w621) -> ("Hout"=w622:u64, "error out"=w623:errorcluster)  [unwired: 1 out]
            n344 = call "SCStopCOC.vi"("error in (no error)"=w623, "Stop mode"=0, "Handle"=w622) -> ("error out"=w616:errorcluster, "Hout"=w617:u64)
          }
          frame #2 {
            n345 = local write "cam_con?"(TRUE ("cam_con?")) -> ()
          }
        }
        n346 = Dequeue Element(queue=w613) -> (queue out=w609:refnum<queue>)  [unwired: 2 in, 3 out]
        n347 = Enqueue Element At Opposite End(queue=w609, element="set") -> ()  [unwired: 2 in, 3 out]
        n348 = call-poly <vilib>:"DAQmx Create Virtual Channel.vi"("lines"=tag "Dev2/port0/line7") -> ("task out"=w603:refnum<k21>)  [unwired: 13 in, 1 out]
      }
      frame "set" {
        n349 = Dequeue Element(queue=w645) -> ()  [unwired: 2 in, 4 out]
        n350 = call "SCStopCOC.vi"("error in (no error)"=w648, "Stop mode"=0, "Handle"=w649) -> ("error out"=w664:errorcluster, "Hout"=w663:u64)
        n351 = Bundle By Name(cluster=cluster{"Delay":dbl, "Exposure ":dbl} {"Delay"=0.0, "Exposure "=0.0} ("Delay and exposure"), "Exposure"="exposure [ms]") -> (w642:cluster{"Delay":dbl, "Exposure ":dbl})
        n352 = Bundle By Name(cluster=T7 {"Camera type"=0, "Operating mode\nHP & QE / HS & DiCam Pro "=0, "Frame trigger \n(High Performance and QE only)"=0, "Sequence trigger"=0, "Low Light\n(QE only)"=FALSE, "Gain"=FALSE, "Horzontal\nbinning"=0, "Vertical\nbinning "=0, "ROI Left"=1, "ROI Right"=20, "ROI Top"=1, "ROI Bottom"=15} ("Camera controls"), "Operating mode\nHP & QE / HS & DiCam Pro"="Operating mode\nHP & QE / HS & DiCam Pro", "Horzontal\nbinning"="binning", "Vertical\nbinning"="binning", "ROI Left"="ROI Left", "ROI Right"="ROI Right", "ROI Top"="ROI Top", "ROI Bottom"="ROI Bottom", "Gain"="gain", "Frame trigger \n(High Performance and QE only)"="Frame trigger \n(High Performance and QE only)") -> (w659:T7)
        n353 = call "New delay and exposure forma.vi"("Operating mode\nHP & QE / HS & DiCam Pro"="Operating mode\nHP & QE / HS & DiCam Pro", "Delay and exposure"=w642) -> ("Output table"=w660:string)  [unwired: 3 in]
        n354 = call "SCSetCoC.vi"("error in (no error)"=w664, "Delay and exposure table"=w660, "Camera controls"=w659, "Handle"=w663) -> ("error out"=w652:errorcluster, "Hout"=w651:u64)  [unwired: 1 out]
        n355 = call "SCGetImageSize.vi"("Handle"=w651, "error in (no error)"=w652) -> ("Hout"=w650:u64, "error out"=w634:errorcluster, "Horizontal size"=w639:i32, "Vertical size"=w638:i32)  [unwired: 2 out]
        n356 = Greater?(x=w639, y=w638) -> (0:w640:bool)
        n357 = Initialize Array(u16 0 ("dimension size"), w638, w639) -> (w632:u16[][])
        n358 = call "SCRun.vi"("error in (no error)"=w634, "Run mode"=0, "Handle"=w650) -> ("error out"=w647:errorcluster, "Hout"=w646:u64)  [unwired: 1 out]
        n359 = Select(t=w639, s=w640, f=w638) -> (s? t:f=w637:i32)
        n360 = property on="mainimg" class="IntGraph (strict)"("XScale.Maximum"=w637, "YScale.Maximum"=w637) -> ()  [unwired: 2 in, 2 out]
      }
      frame "bench" {
        n361 = Dequeue Element(queue=w675) -> ()  [unwired: 2 in, 4 out]
        n362 = call "SCStopCOC.vi"("error in (no error)"=w677, "Stop mode"=0, "Handle"=w685) -> ("error out"=w669:errorcluster, "Hout"=w670:u64)
        n363 = while {
          tunnel: w671 -> [w701]
          tunnel: w670 -> [w700]
          tunnel: w669 -> [w691]
          shift-right: [w697] -> _
          shift-left: _ -> [w696]
          tunnel: [w693] -> w668
          tunnel: [w692] -> w667
          tunnel: w666 -> [w688]
          tunnel: [w687] -> w665
          stop <- "stop" stop-if-true
          n364 = call "wait4trig.vi"("error in"=w691, "task/channels in"=w688) -> ("error out"=w690:errorcluster, "voltage out"=→"voltage out":dbl, "task out"=w687:refnum<k21>)  [unwired: 7 in]
          n365 = call "SCRun.vi"("error in (no error)"=w690, "Run mode"=4, "Handle"=w700) -> ("error out"=w702:errorcluster, "Hout"=w703:u64)  [unwired: 1 out]
          n366 = call <vilib>:"High Resolution Relative Seconds.vi"() -> ("relative seconds"=w697:dbl)
          n367 = call "grabimg.vi"("array in"=w701, "error in"=w702, "Hin"=w703) -> ("error out"=w692:errorcluster, "imgdata"=w699:i32[][], "Hout"=w693:u64)  [unwired: 6 in]
          n368 = To Double Precision Float(number=w699) -> (double precision float=→"sideimg 2":dbl[][])
          n369 = Subtract(x=w697, y=w696) -> (x-y=w694:dbl)
          "x/y" <- w694
          n370 = Reciprocal(x=w694) -> (1/x=→"1/x":dbl)
        }
        n371 = call "SCStopCOC.vi"("error in (no error)"=w667, "Stop mode"=0, "Handle"=w668) -> ("error out"=w672:errorcluster, "Hout"=w673:u64)
        n372 = call "SCRun.vi"("error in (no error)"=w672, "Run mode"=0, "Handle"=w673) -> ("error out"=w682:errorcluster, "Hout"=w681:u64)  [unwired: 1 out]
      }
      frame "release" {
        n373 = Dequeue Element(queue=w715) -> ()  [unwired: 2 in, 4 out]
        n374 = flat-sequence {
          tunnel: w713 -> [w717]
          tunnel: [w716] -> w710
          tunnel: [w719] -> w711
          tunnel: w710 -> [w719]
          frame #0 {
            n375 = call "SCCloseBoard.vi"("Handle"=w717) -> ("error out"=w716:errorcluster)  [unwired: 1 in, 2 out]
          }
          frame #1 {
            n376 = local write "cam_con?"(FALSE ("cam_con?")) -> ()
          }
        }
        n377 = call <vilib>:"DAQmx Clear Task.vi"("task in"=w706) -> ()  [unwired: 14 in, 1 out]
      }
      frame "close" {
        n378 = Release Queue(queue=w728) -> ()  [unwired: 2 in, 3 out]
      }
      frame "idle", Default {
        n379 = call "grabimg.vi"("array in"=w769, "error in"=w775, "Hin"=w776) -> ("error out"=w774:errorcluster, "imgdata"=w772:i32[][], "Hout"=w773:u64)  [unwired: 6 in]
        n380 = local read "lower threshold"() -> (w767:i32)
        n381 = case shown="True" "cam_dark?" {
          tunnel: w778 -> [_ w801]
          tunnel: [w798 w800] -> w768
          tunnel: w772 -> [w798 w799]
          frame False {
          }
          frame True {
            n382 = Subtract(x=w799, y=w801) -> (x-y=w800:dbl[][])
          }
        }
        n383 = call "filtr_b.vi"("threshold"=w767, "input array"=w768) -> ("output array"=w759:dbl[][])  [unwired: 9 in]
        n384 = call <vilib>:"High Resolution Relative Seconds.vi"() -> ("relative seconds"=w783:dbl)
        n385 = Subtract(x=w783, y=w782) -> (x-y=w781:dbl)
        n386 = Array Size(array=w759) -> (size(s)=w758:i32[])
        n387 = Reciprocal(x=w781) -> (1/x=→"cam_fps":dbl)
        n388 = Index Array(array=w758) -> (element #1=w753:i32, element #2=w752:i32)  [unwired: 2 in]
        n389 = Subtract(x=w744, y=w743) -> (x-y=w742:i32)
        n390 = Less Or Equal?(x="pics2avg", y=w742) -> (x <= y?=w765:bool)
        n391 = And(x="reset every n pics", y=w765) -> (x .and. y?=w763:bool)
        n392 = Not(x=w763) -> (.not. x?=w762:bool)
        n393 = call-poly <vilib>:"Ramp Pattern.vi"("start"=0.0, "end"=w753, "samples"=w753) -> ("Ramp Pattern"=w748:dbl[])  [unwired: 7 in, 1 out]
        n394 = call-poly <vilib>:"Ramp Pattern.vi"("start"=0.0, "end"=w752, "samples"=w752) -> ("Ramp Pattern"=w749:dbl[])  [unwired: 7 in, 1 out]
        n395 = property on="mainimg" class="IntGraph (strict)"() -> ("CrsrLis"=w741:T5)  [unwired: 2 in, 2 out]
        n396 = And(x="cam_liveavg", y=w762) -> (x .and. y?=w760:bool)
        n397 = case shown="False" w760 {
          tunnel: w759 -> [w788 w794]
          tunnel: [w788 w791] -> w736
          tunnel: w771 -> [_ w796]
          tunnel: w744 -> [w789 _]
          tunnel: [w789 w797] -> w770
          tunnel: w743 -> [_ w797]
          tunnel: w742 -> [_ w790]
          frame False {
          }
          frame True {
            n398 = Multiply(x=w796, y=w790) -> (x*y=w795:dbl[][])
            n399 = Increment(x=w790) -> (x+1=w792:i32)
            n400 = Add(x=w795, y=w794) -> (x+y=w793:dbl[][])
            n401 = Divide(x=w793, y=w792) -> (x/y=w791:dbl[][])
          }
        }
        "mainimg" <- w736
        n402 = Index Array(array=w741) -> (element #1=w739:T8, element #2=w740:T8)  [unwired: 2 in]
        n403 = Unbundle By Name(w739) -> ("Position.X"=w733:dbl, "Position.Y"=w735:dbl)
        n404 = Unbundle By Name(w740) -> ("Position.X"=w737:dbl, "Position.Y"=w738:dbl)
        n405 = Array Max & Min(array=w736) -> (max value=→"max":dbl)  [unwired: 3 out]
        n406 = Subtract(x=w738, y=w735) -> (x-y=w734:dbl)
        n407 = Subtract(x=w737, y=w733) -> (x-y=w732:dbl)
        n408 = Array Subset(array=w736, index (row)=w735, length (row)=w734) -> (w747:dbl[][])  [unwired: 2 in]
        n409 = Array Subset(array=w736, index (col)=w733, length (col)=w732) -> (w745:dbl[][])  [unwired: 2 in]
        n410 = Array Subset(array=w736, index (row)=w735, length (row)=w734, index (col)=w733, length (col)=w732) -> (w731:dbl[][])
        n411 = Transpose 2D Array(2D array=w747) -> (transposed array=w746:dbl[][])
        n412 = Add Array Elements(numeric array=w731) -> (sum=→"sum" →"Waveform Chart":dbl)
        n413 = for {
          tunnel: w745 -> [w785] mode=indexing
          tunnel: [w784] -> w755 mode=indexing
          n414 = Add Array Elements(numeric array=w785) -> (sum=w784:dbl)
        }
        n415 = for {
          tunnel: w746 -> [w787] mode=indexing
          tunnel: [w786] -> w754 mode=indexing
          n416 = Add Array Elements(numeric array=w787) -> (sum=w786:dbl)
        }
        n417 = Bundle("Ramp Pattern"=w749, w754) -> (→"G2 X":cluster{"Ramp Pattern":dbl[], dbl[]})  [unwired: 1 in]
        n418 = Bundle(w755, "Ramp Pattern"=w748) -> (→"G2 Y":cluster{dbl[], "Ramp Pattern":dbl[]})  [unwired: 1 in]
      }
      frame "dark" {
        n419 = Dequeue Element(queue=w816) -> ()  [unwired: 2 in, 4 out]
        n420 = Array Size(array=w813) -> (size(s)=w812:i32[])
        n421 = Index Array(array=w812) -> (element #1=w811:i32, element #2=w810:i32)  [unwired: 2 in]
        n422 = Initialize Array(0.0 ("element"), w811, w810) -> (w808:dbl[][])
        n423 = for {
          N: "dark avg" -> [_]
          tunnel: w818 -> [w826]
          tunnel: w817 -> [w825]
          tunnel: [w824] -> w815
          tunnel: w813 -> [w823]
          tunnel: [w822] -> w814
          shift-right: [w819] -> w806
          shift-left: w808 -> [w820]
          n424 = call "grabimg.vi"("array in"=w823, "error in"=w825, "Hin"=w826) -> ("error out"=w824:errorcluster, "imgdata"=w821:i32[][], "Hout"=w822:u64)  [unwired: 6 in]
          n425 = Add(x=w821, y=w820) -> (x+y=w819:dbl[][])
        }
        n426 = Divide(x=w806, y="dark avg") -> (x/y=w807:dbl[][])
      }
      frame "snap" {
        w830 = 0
        n427 = Dequeue Element(queue=w849) -> ()  [unwired: 2 in, 4 out]
        n428 = local read "cam_dark?"() -> (w848:bool)
        n429 = local read "averages"() -> (w843:i32)
        n430 = To Double Precision Float(number=w834) -> (double precision float=w833:dbl[][])
        n431 = Equal To 0?(x="aq.mode") -> (x = 0?=w836:bool)
        n432 = Get Date/Time In Seconds() -> (seconds since 1Jan1904=w839:timestamp)
        n433 = for {
          N: w843 -> [w868]
          shift-right: [w886] -> w844
          shift-left: w846 -> [w888]
          shift-right: [w873] -> w842
          shift-left: w845 -> [w887]
          tunnel: w848 -> [w884]
          tunnel: w847 -> [w883]
          tunnel: w834 -> [w882]
          tunnel: w839 -> [w878]
          tunnel: w836 -> [w861]
          shift-right: [w869] -> w827
          shift-left: w833 -> [w870]
          shift-right: [w856] -> w829
          shift-left: w833 -> [w860]
          shift-right: [w859] -> w831
          shift-left: w832 -> [w855]
          shift-right: [w853] -> _
          shift-left: w830 -> [w854]
          shift-right: [w852] -> _
          shift-left: w830 -> [w850]
          i -> [w858]
          stop <- "abort acq." stop-if-true
          n434 = call "grabimg.vi"("array in"=w882, "error in"=w887, "Hin"=w888) -> ("error out"=w873:errorcluster, "imgdata"=w885:i32[][], "Hout"=w886:u64)  [unwired: 6 in]
          n435 = local read "lower threshold"() -> (w864:i32)
          n436 = Increment(x=w858) -> (x+1=w866:i32)
          "acq. imgs" <- w866
          n437 = Get Date/Time In Seconds() -> (seconds since 1Jan1904=w881:timestamp)
          n438 = case shown="True" w884 {
            tunnel: w885 -> [w979 w982]
            tunnel: w883 -> [_ w981]
            tunnel: [w979 w980] -> w863
            frame False {
            }
            frame True {
              n439 = Subtract(x=w982, y=w981) -> (x-y=w980:dbl[][])
            }
          }
          n440 = Divide(x=w866, y=w868) -> (x/y=→"snap_prog":dbl)
          n441 = Subtract(x=w881, y=w878) -> (x-y=w880:dbl)
          n442 = call "filtr_b.vi"("threshold"=w864, "input array"=w863) -> ("output array"=w862:dbl[][])  [unwired: 9 in]
          n443 = Divide(x=w880, y=w858) -> (x/y=w876:dbl)
          n444 = Multiply(x=w876, y=w868) -> (x*y=w879:dbl)
          n445 = Reciprocal(x=w876) -> (1/x=w875:dbl)
          n446 = case shown="True" "count?" {
            tunnel: w862 -> [w968 w970]
            tunnel: "e-size" -> [_ w972]
            tunnel: w864 -> [_ w971]
            tunnel: [w968 w969] -> w857
            frame False {
            }
            frame True {
              n447 = Array Size(array=w970) -> (size(s)=w974:i32[])
              n448 = call "findr.vi"("thresh"=w971, "esize"=w972, "inp array"=w970) -> ("locs"=w973:i32[][])  [unwired: 8 in]
              n449 = Index Array(array=w974) -> (element #1=w976:i32, element #2=w975:i32)  [unwired: 2 in]
              n450 = call "drawe.vi"("Ysize"=w976, "Xsize"=w975, "pos array"=w973) -> ("img out"=w969:i32[][])  [unwired: 8 in]
            }
          }
          n451 = case shown="True" "Enable Chopping" {
            tunnel: w870 -> [w896 w923]
            tunnel: [w892 w922] -> w869
            tunnel: w861 -> [w891 w921]
            tunnel: w860 -> [w889 w920]
            tunnel: [w893 w919] -> w859
            tunnel: w857 -> [w897 w917]
            tunnel: [w889 w915] -> w856
            tunnel: w855 -> [w893 w914]
            tunnel: w854 -> [w895 w913]
            tunnel: [w894 w912] -> w853
            tunnel: [w890 w911] -> w852
            tunnel: w850 -> [w890 w910]
            frame False {
              n452 = case shown="True" w891 {
                tunnel: w897 -> [w900 w908]
                tunnel: w895 -> [w899 w907]
                tunnel: w896 -> [w902 w906]
                tunnel: [w901 w904] -> w892
                tunnel: [w898 w903] -> w894
                frame False {
                  n453 = Add(x=w900, y=w902) -> (x+y=w901:dbl[][])
                  n454 = Increment(x=w899) -> (x+1=w898:i32)
                }
                frame True {
                  n455 = Multiply(x=w906, y=w907) -> (x*y=w909:dbl[][])
                  n456 = Increment(x=w907) -> (x+1=w903:i32)
                  n457 = Add(x=w908, y=w909) -> (x+y=w905:dbl[][])
                  n458 = Divide(x=w905, y=w903) -> (x/y=w904:dbl[][])
                }
              }
            }
            frame True {
              n459 = flat-sequence {
                tunnel: [w925] -> w919
                tunnel: [w924] -> w918
                tunnel: w917 -> [w927]
                tunnel: [w927] -> w916
                tunnel: [w926] -> _
                tunnel: w914 -> [w926]
                frame #0 {
                  n460 = call-poly <vilib>:"DAQmx Read.vi"("task/channels in"=w926) -> ("task out"=w925:refnum<k21>, "data"=w924:bool)  [unwired: 12 in, 1 out]
                  "Pump Laser" <- w924
                }
              }
              n461 = case shown="False" w918 {
                tunnel: w921 -> [w933 _]
                tunnel: w920 -> [w932 w947]
                tunnel: [w931 w947] -> w915
                tunnel: w916 -> [w930 _]
                tunnel: w910 -> [w929 w946]
                tunnel: [w928 w946] -> w911
                frame False {
                  n462 = case shown="True" w933 {
                    tunnel: w930 -> [w936 w944]
                    tunnel: w929 -> [w935 w943]
                    tunnel: w932 -> [w938 w942]
                    tunnel: [w937 w940] -> w931
                    tunnel: [w934 w939] -> w928
                    frame False {
                      n463 = Add(x=w936, y=w938) -> (x+y=w937:dbl[][])
                      n464 = Increment(x=w935) -> (x+1=w934:i32)
                    }
                    frame True {
                      n465 = Multiply(x=w942, y=w943) -> (x*y=w945:dbl[][])
                      n466 = Increment(x=w943) -> (x+1=w939:i32)
                      n467 = Add(x=w944, y=w945) -> (x+y=w941:dbl[][])
                      n468 = Divide(x=w941, y=w939) -> (x/y=w940:dbl[][])
                    }
                  }
                }
                frame True {
                }
              }
              n469 = case shown="True" w918 {
                tunnel: w923 -> [w949 w955]
                tunnel: [w949 w954] -> w922
                tunnel: w921 -> [_ w953]
                tunnel: w916 -> [_ w952]
                tunnel: w913 -> [w948 w951]
                tunnel: [w948 w950] -> w912
                frame False {
                }
                frame True {
                  n470 = case shown="True" w953 {
                    tunnel: w952 -> [w958 w966]
                    tunnel: w951 -> [w957 w965]
                    tunnel: w955 -> [w960 w964]
                    tunnel: [w959 w962] -> w954
                    tunnel: [w956 w961] -> w950
                    frame False {
                      n471 = Add(x=w958, y=w960) -> (x+y=w959:dbl[][])
                      n472 = Increment(x=w957) -> (x+1=w956:i32)
                    }
                    frame True {
                      n473 = Multiply(x=w964, y=w965) -> (x*y=w967:dbl[][])
                      n474 = Increment(x=w965) -> (x+1=w961:i32)
                      n475 = Add(x=w966, y=w967) -> (x+y=w963:dbl[][])
                      n476 = Divide(x=w963, y=w961) -> (x/y=w962:dbl[][])
                    }
                  }
                }
              }
            }
          }
          "Pics NL" <- w852
          "Pics L" <- w853
          n477 = Add(x=w879, y=w878) -> (x+y=→"ETA":timestamp)
          n478 = local write "cam_fps"(w875) -> ()
          n479 = local write "mainimg"(w862) -> ()
          n480 = Transpose 2D Array(2D array=w862) -> (transposed array=w874:dbl[][])
          n481 = for {
            tunnel: w874 -> [w978] mode=indexing
            tunnel: [w977] -> _ mode=indexing
            n482 = Add Array Elements(numeric array=w978) -> (sum=w977:dbl)
          }
          n483 = local write "sideimg 2"(w856) -> ()
          n484 = local write "sideimg"(w869) -> ()
        }
        n485 = Build Array(w827, w829) -> (w828:dbl[][][])
        n486 = Enqueue Element(queue=w838, element=w828, error in (no error)=w842) -> (error out=w835:errorcluster)  [unwired: 1 in, 2 out]
      }
      frame "suspend" {
        n487 = Dequeue Element(queue=w991) -> ()  [unwired: 2 in, 4 out]
      }
    }
    "cam_error" <- w592
  }
  n488 = while {
    tunnel: w10 -> [w997]
    tunnel: w13 -> [w996]
    tunnel: w3 -> [w995]
    tunnel: w24 -> [w994]
    tunnel: w2 -> [w992]
    tunnel: w11 -> [w993]
    stop <- w998 stop-if-true
    n489 = event shown="[21] \"ESP_dest_t\": Value Change" {
      selector: _ -> [_ _ _ _ _ _ _ _ _ _ _ _ _ _ _ _ _ _ _ _ _ _ _ _ _ _ _]
      dyn-events: _ -> [_ _ _ _ _ _ _ _ _ _ _ _ _ _ _ _ _ _ _ _ _ _ _ _ _ _ _]
      timeout: _ -> [_ _ _ _ _ _ _ _ _ _ _ _ _ _ _ _ _ _ _ _ _ _ _ _ _ _ _]
      tunnel: [_ TRUE _ _ _ _ _ _ _ _ _ _ _ _ _ _ _ _ _ _ _ _ _ _ _ _ _] -> w998
      tunnel: w997 -> [_ w1011 w1014 _ _ _ _ _ w1040 w1042 _ _ _ _ _ _ _ _ _ _ _ _ _ _ _ _ w1149]
      tunnel: w996 -> [_ w1010 _ w1018 _ _ _ _ _ _ _ _ _ _ _ _ _ w1075 _ w1087 _ _ _ _ _ _ _]
      tunnel: w995 -> [_ w1009 _ _ w1024 _ _ _ _ _ _ _ _ _ w1063 _ w1067 _ _ _ _ _ _ _ _ _ _]
      tunnel: w994 -> [_ w1008 _ _ _ w1030 w1036 w1037 _ _ _ _ _ _ _ _ _ _ _ _ _ _ _ _ _ _ _]
      tunnel: w993 -> [_ w1002 _ _ _ _ _ _ _ _ _ _ _ _ _ _ _ _ _ _ _ _ _ _ _ _ _]
      tunnel: w992 -> [_ w1001 _ _ _ _ _ _ _ _ w1044 w1046 w1047 _ _ w1065 _ _ _ _ _ _ _ _ _ w1148 _]
      event Timeout {
        n490 = event-data() -> ()  [unwired: 1 in, 1 out]
        n491 = call-poly <vilib>:"Read Delimited Spreadsheet.vi"() -> ("all rows"=w999:string[][])  [unwired: 10 in, 5 out]
        n492 = local write "delay table [fs]"(w999) -> ()
      }
      event "main_close": Value Change {
        w1000 = "close" ("element")
        w1007 = "release" ("element")
        n493 = event-data() -> ()  [unwired: 1 in, 1 out]
        n494 = Release Queue(queue=w1002) -> ()  [unwired: 2 in, 3 out]
        n495 = Enqueue Element(queue=w1011, element=w1007) -> (queue out=w1006:refnum<queue>)  [unwired: 2 in, 2 out]
        n496 = Enqueue Element(queue=w1010, element=w1007) -> (queue out=w1005:refnum<queue>)  [unwired: 2 in, 2 out]
        n497 = Enqueue Element(queue=w1009, element=w1007) -> (queue out=w1004:refnum<queue>)  [unwired: 2 in, 2 out]
        n498 = Enqueue Element(queue=w1008, element=w1007) -> (queue out=w1003:refnum<queue>)  [unwired: 2 in, 2 out]
        n499 = Enqueue Element(queue=w1006, element=w1000) -> ()  [unwired: 2 in, 3 out]
        n500 = Enqueue Element(queue=w1005, element=w1000) -> ()  [unwired: 2 in, 3 out]
        n501 = Enqueue Element(queue=w1004, element=w1000) -> ()  [unwired: 2 in, 3 out]
        n502 = Enqueue Element(queue=w1003, element=w1000) -> ()  [unwired: 2 in, 3 out]
        n503 = Enqueue Element(queue=w1001, element=w1000) -> ()  [unwired: 2 in, 3 out]
      }
      event "cam_release", "cam_init": Value Change {
        n504 = event-data() -> ()  [unwired: 1 in, 2 out]
        n505 = Select(t="init" ("name (unnamed)"), s="cam_init", f="release" ("name (unnamed)")) -> (s? t:f=w1013:string)
        n506 = Enqueue Element(queue=w1014, element=w1013) -> ()  [unwired: 2 in, 3 out]
      }
      event "ESP_release", "ESP_init": Value Change {
        n507 = event-data() -> ()  [unwired: 1 in, 2 out]
        n508 = Select(t="init" ("name (unnamed)"), s="ESP_init", f="release" ("name (unnamed)")) -> (s? t:f=w1022:string)
        n509 = Enqueue Element(queue=w1018, element=w1022) -> ()  [unwired: 2 in, 3 out]
      }
      event "manip_init", "manip_release": Value Change {
        n510 = event-data() -> ()  [unwired: 1 in, 2 out]
        n511 = Flush Queue(queue=w1024) -> (queue out=w1023:refnum<queue>)  [unwired: 1 in, 2 out]
        n512 = Select(t="init" ("name (unnamed)"), s="manip_init", f="release" ("name (unnamed)")) -> (s? t:f=w1026:string)
        n513 = Enqueue Element(queue=w1023, element=w1026) -> ()  [unwired: 2 in, 3 out]
      }
      event "phoib_release", "phoib_init": Value Change {
        n514 = event-data() -> ()  [unwired: 1 in, 2 out]
        n515 = Flush Queue(queue=w1030) -> (queue out=w1029:refnum<queue>)  [unwired: 1 in, 2 out]
        n516 = Select(t="init" ("name (unnamed)"), s="phoib_init", f="release" ("name (unnamed)")) -> (s? t:f=w1032:string)
        n517 = Enqueue Element(queue=w1029, element=w1032) -> ()  [unwired: 2 in, 3 out]
      }
      event "phoib_standby": Value Change {
        n518 = event-data() -> ()  [unwired: 1 in, 2 out]
        n519 = Enqueue Element(queue=w1036, element="standby") -> ()  [unwired: 2 in, 3 out]
      }
      event "phoib_set": Value Change {
        n520 = event-data() -> ()  [unwired: 1 in, 2 out]
        n521 = Enqueue Element(queue=w1037, element="set") -> ()  [unwired: 2 in, 3 out]
      }
      event "cam_dark": Value Change {
        n522 = event-data() -> ()  [unwired: 1 in, 2 out]
        n523 = Enqueue Element(queue=w1040, element="dark") -> ()  [unwired: 2 in, 3 out]
      }
      event "ROI Left", "ROI Right", "ROI Top", "ROI Bottom", "exposure [ms]", "binning", "gain": Value Change {
        n524 = event-data() -> ()  [unwired: 1 in, 1 out]
        n525 = Enqueue Element(queue=w1042, element="set") -> ()  [unwired: 2 in, 3 out]
      }
      event "cam_saveimg": Value Change {
        n526 = event-data() -> ()  [unwired: 1 in, 1 out]
        n527 = Enqueue Element(queue=w1044, element="single") -> ()  [unwired: 2 in, 3 out]
      }
      event "delscan_go": Value Change {
        n528 = event-data() -> ()  [unwired: 1 in, 1 out]
        n529 = Enqueue Element(queue=w1046, element="GO") -> ()  [unwired: 2 in, 3 out]
      }
      event "delscan_go 2": Value Change {
        n530 = event-data() -> ()  [unwired: 1 in, 1 out]
        n531 = Enqueue Element(queue=w1047, element="delay_chop") -> ()  [unwired: 2 in, 3 out]
      }
      event "Move Abs": Value Change {
        n532 = event-data() -> ()  [unwired: 1 in, 1 out]
      }
      event "ManipRel +", "ManipRel -": Value Change {
        n533 = event-data() -> ()  [unwired: 1 in, 2 out]
        n534 = Negate(x="manip_deltas") -> (-x=w1051:dbl[])
        n535 = Select(t="manip_deltas", s="ManipRel +", f=w1051) -> (s? t:f=w1049:dbl[])
        n536 = Index Array(array=w1049) -> (element #1=w1055:dbl, element #2=w1056:dbl, element #3=w1057:dbl, element #4=w1058:dbl, element #5=w1059:dbl, element #6=w1060:dbl)  [unwired: 6 in]
        n537 = Format Into String(format string="%g_%g_%g_%g_%g_%g", w1055, w1056, w1057, w1058, w1059, w1060) -> (resulting string=w1062:string)  [unwired: 2 in, 1 out]
        n538 = Concatenate Strings("relative:" ("string"), w1062) -> (w1053:string)
        n539 = Enqueue Element(queue=w1063, element=w1053) -> ()  [unwired: 2 in, 3 out]
      }
      event "Optimize": Value Change {
        n540 = event-data() -> ()  [unwired: 1 in, 6 out]
        n541 = Enqueue Element(queue=w1065, element="manip") -> ()  [unwired: 2 in, 3 out]
      }
      event "stop manip": Value Change {
        n542 = event-data() -> ()  [unwired: 1 in, 1 out]
        n543 = Enqueue Element(queue=w1067, element="stop") -> ()  [unwired: 2 in, 3 out]
      }
      event "ESP_go": Value Change {
        w1069 = ":" ("string")
        n544 = event-data() -> ()  [unwired: 1 in, 1 out]
        n545 = local read "ESP Axis"() -> (w1068:i32)
        n546 = Number To Decimal String(number=w1068) -> (decimal integer string=w1071:string)  [unwired: 1 in]
        n547 = Number To Fractional String(number="ESP_dest") -> (F-format string=w1070:string)  [unwired: 3 in]
        n548 = Concatenate Strings("abs:" ("string"), w1071, w1069, w1070, w1069) -> (w1074:string)
        n549 = Enqueue Element(queue=w1075, element=w1074) -> ()  [unwired: 2 in, 3 out]
      }
      event "ESP_set_t0": Value Change {
        n550 = event-data() -> ()  [unwired: 1 in, 1 out]
        n551 = Current VI's Path() -> (path=w1081:path)
        n552 = Strip Path(path=w1081) -> (stripped path=w1077:path)  [unwired: 1 out]
        n553 = Strip Path(path=w1077) -> (stripped path=w1076:path)  [unwired: 1 out]
        n554 = local read "ESP_pos"() -> (w1079:dbl)
        "ESP_t0" <- w1079
        n555 = Number To Fractional String(number=w1079) -> (F-format string=w1078:string)  [unwired: 3 in]
        n556 = Build Path(base path=w1076, name or relative path="t0.txt") -> (appended path=w1080:path)
        n557 = Write to Text File(file (use dialog)=w1080, text=w1078) -> ()  [unwired: 2 in, 3 out]
      }
      event "ESP_+", "ESP_-": Value Change {
        n558 = event-data() -> ()  [unwired: 1 in, 6 out]
        n559 = Negate(x="ESP_delta") -> (-x=w1090:dbl)
        n560 = Select(t="ESP_delta", s="ESP_+", f=w1090) -> (s? t:f=w1088:dbl)
        n561 = Number To Decimal String(number="ESP Axis") -> (decimal integer string=w1085:string)  [unwired: 1 in]
        n562 = Number To Fractional String(number=w1088) -> (F-format string=w1083:string)  [unwired: 3 in]
        n563 = Concatenate Strings("rel:" ("string"), w1085, ":" ("string"), w1083) -> (w1093:string)
        n564 = Enqueue Element(queue=w1087, element=w1093) -> ()  [unwired: 2 in, 3 out]
      }
      event "ESP_dest": Value Change {
        n565 = event-data() -> ()  [unwired: 1 in, 6 out]
        n566 = local read "ESP_dest"() -> (w1097:dbl)
        n567 = local read "ESP_t0"() -> (w1096:dbl)
        n568 = call "mm2time.vi"("fs?"=TRUE ("fs[1]/ps[0]"), "Offset (mm)"=w1096, "distance (mm)"=w1097) -> ("time in fs/ps seconds"=w1094:dbl)
        n569 = local write "ESP_dest_t"(w1094) -> ()
      }
      event "ESP_dest_t": Value Change {
        n570 = event-data() -> ()  [unwired: 1 in, 1 out]
        n571 = local read "ESP_t0"() -> (w1100:dbl)
        n572 = call "time2mm.vi"("fs[1]/ps[0]"=TRUE, "Offset (mm)"=w1100, "time"="ESP_dest_t") -> ("position (mm)"=w1098:dbl)
        n573 = local write "ESP_dest"(w1098) -> ()
      }
      event "load delay table": Value Change {
        n574 = event-data() -> ()  [unwired: 1 in, 6 out]
        n575 = call-poly <vilib>:"Read Delimited Spreadsheet.vi"() -> ("all rows"=w1103:string[][])  [unwired: 10 in, 5 out]
        n576 = local read "binning"() -> (w1110:u16)
        n577 = local write "delay table [fs]"(w1103) -> ()
        n578 = local read "delscan_iters"() -> (w1104:u32)
        n579 = local read "time / step"() -> (w1113:dbl)
        n580 = Array Size(array=w1103) -> (size(s)=w1114:i32[])
        n581 = Index Array(array=dbl[] [8.79, 2.2, 0.553, 0.138], index=w1110) -> (element=w1108:dbl)
        n582 = Index Array(array=w1114) -> (element #1=w1102:i32)  [unwired: 2 in, 1 out]
        n583 = Multiply(x=w1104, y=w1102) -> (x*y=w1107:u32)
        n584 = Multiply(x=w1102, y=w1108) -> (x*y=w1109:dbl)
        n585 = Multiply(x=w1107, y=w1113) -> (x*y=w1112:dbl)
        n586 = Increment(x=w1107) -> (x+1=w1106:u32)
        n587 = Multiply(x=w1106, y=w1108) -> (x*y=w1105:dbl)
        n588 = local write "delaypoints"(w1102) -> ()
        n589 = local write "total steps"(w1107) -> ()
        n590 = local write "duration [HH:MM:SS]"(w1112) -> ()
        n591 = local write "RAM [MB]"(w1109) -> ()
        n592 = local write "disk [MB]"(w1105) -> ()
      }
      event "delay table [fs]", "delscan_iters": Value Change {
        n593 = event-data() -> ()  [unwired: 1 in, 6 out]
        n594 = local read "binning"() -> (w1123:u16)
        n595 = local read "delay table [fs]"() -> (w1127:string[][])
        n596 = local read "delscan_iters"() -> (w1117:u32)
        n597 = local read "time / step"() -> (w1125:dbl)
        n598 = Array Size(array=w1127) -> (size(s)=w1126:i32[])
        n599 = Index Array(array=dbl[] [8.79, 2.2, 0.553, 0.138], index=w1123) -> (element=w1121:dbl)
        n600 = Index Array(array=w1126) -> (element #1=w1115:i32)  [unwired: 2 in, 1 out]
        n601 = Multiply(x=w1117, y=w1115) -> (x*y=w1120:u32)
        n602 = Multiply(x=w1115, y=w1121) -> (x*y=w1122:dbl)
        n603 = Multiply(x=w1120, y=w1125) -> (x*y=w1124:dbl)
        n604 = Increment(x=w1120) -> (x+1=w1119:u32)
        n605 = Multiply(x=w1119, y=w1121) -> (x*y=w1118:dbl)
        n606 = local write "delaypoints"(w1115) -> ()
        n607 = local write "total steps"(w1120) -> ()
        n608 = local write "duration [HH:MM:SS]"(w1124) -> ()
        n609 = local write "RAM [MB]"(w1122) -> ()
        n610 = local write "disk [MB]"(w1118) -> ()
      }
      event "generate delay table": Value Change {
        n611 = event-data() -> ()  [unwired: 1 in, 1 out]
        n612 = call "getdelaypoints.vi"("delscan_stepsize"="delscan_stepsize", "delscan_end"="delscan_end", "delscan_start"="delscan_start") -> ("delaypoints"=w1143:dbl[])
        n613 = Number To Fractional String(number=w1143) -> (F-format string=w1142:string[])  [unwired: 3 in]
        n614 = Build Array(w1142) -> (w1141:string[][])
        n615 = Transpose 2D Array(2D array=w1141) -> (transposed array=w1128:string[][])
        n616 = local write "delay table [fs]"(w1128) -> ()
        n617 = local read "binning"() -> (w1137:u16)
        n618 = local read "delscan_iters"() -> (w1131:u32)
        n619 = local read "time / step"() -> (w1139:dbl)
        n620 = Array Size(array=w1128) -> (size(s)=w1140:i32[])
        n621 = Index Array(array=dbl[] [8.79, 2.2, 0.553, 0.138], index=w1137) -> (element=w1135:dbl)
        n622 = Index Array(array=w1140) -> (element #1=w1129:i32)  [unwired: 2 in, 1 out]
        n623 = Multiply(x=w1131, y=w1129) -> (x*y=w1134:u32)
        n624 = Multiply(x=w1129, y=w1135) -> (x*y=w1136:dbl)
        n625 = Multiply(x=w1134, y=w1139) -> (x*y=w1138:dbl)
        n626 = Increment(x=w1134) -> (x+1=w1133:u32)
        n627 = Multiply(x=w1133, y=w1135) -> (x*y=w1132:dbl)
        n628 = local write "delaypoints"(w1129) -> ()
        n629 = local write "total steps"(w1134) -> ()
        n630 = local write "duration [HH:MM:SS]"(w1138) -> ()
        n631 = local write "RAM [MB]"(w1136) -> ()
        n632 = local write "disk [MB]"(w1132) -> ()
      }
      event "mainimg": Cursor Release {
        n633 = event-data() -> ()  [unwired: 1 in, 1 out]
        n634 = Enqueue Element(queue=w1148, element="refresh") -> ()  [unwired: 2 in, 3 out]
      }
      event "dev_bench": Value Change {
        n635 = event-data() -> ()  [unwired: 1 in, 2 out]
        n636 = Enqueue Element(queue=w1149, element="bench") -> ()  [unwired: 2 in, 3 out]
      }
    }
  }
  n637 = while {
    tunnel: w13 -> [w1159]
    shift-right: [w1157] -> _
    shift-left: _ -> [w1155]
    shift-right: [w1156] -> _
    shift-left: _ -> [w1154]
    shift-right: [w1152] -> _
    shift-left: 0 -> [w1153]
    tunnel: w2 -> [w1151]
    stop <- w1158 stop-if-true
    # "ESP"
    n638 = Preview Queue Element(queue=w1159, timeout in ms (-1)=w1153) -> (queue out=w1162:refnum<queue>, element=w1163:string)  [unwired: 1 in, 2 out]
    n639 = Match Pattern(string=w1163, regular expression=":") -> (before substring=w1161:string, after substring=w1160:string)  [unwired: 1 in, 2 out]
    n640 = case shown="\"abs\"" w1161 {
      tunnel: w1162 -> [_ w1174 w1192 w1226 w1227 w1234 w1239]
      tunnel: w1160 -> [_ w1179 w1199 _ _ _ _]
      tunnel: [_ _ _ _ _ TRUE _] -> w1158
      tunnel: [w1166 w1181 w1193 w1224 refnum<visa-resource-name> refnum ("VISA resource name out") w1231 w1238] -> w1157
      tunnel: [w1165 w1182 w1191 w1223 w1229 w1232 w1237] -> w1156
      tunnel: w1155 -> [w1170 w1184 w1197 w1224 w1230 w1231 _]
      tunnel: w1154 -> [w1169 w1183 w1198 w1223 _ w1232 _]
      tunnel: [_ _ _ -1 _ _ _] -> w1152
      tunnel: w1151 -> [_ _ w1190 _ _ _ _]
      frame "idle", Default {
        n641 = local read "ESP Axis"() -> (w1167:i32)
        n642 = local read "ESP_t0"() -> (w1173:dbl)
        n643 = call "Read Actual Position.vi"("error in (no error)"=w1169, "Axis (1)"=w1167, "VISA resource name"=w1170) -> ("error out"=w1165:errorcluster, "Position (units)"=w1168:dbl, "VISA resource name out"=w1166:refnum<visa-resource-name>)  [unwired: 2 in]
        "ESP_pos" <- w1168
        n644 = call "mm2time.vi"("fs?"=TRUE, "Offset (mm)"=w1173, "distance (mm)"=w1168) -> ("time in fs/ps seconds"=→"ESP_delay":dbl)
      }
      frame "rel" {
        n645 = Match Pattern(string=w1179, regular expression=":") -> (before substring=w1178:string, after substring=w1177:string)  [unwired: 1 in, 2 out]
        n646 = Dequeue Element(queue=w1174) -> ()  [unwired: 2 in, 4 out]
        n647 = Decimal String To Number(string=w1178) -> (number=w1176:i32)  [unwired: 2 in, 1 out]
        n648 = Fract/Exp String To Number(string=w1177) -> (number=w1175:dbl)  [unwired: 3 in, 1 out]
        n649 = call "Move Relative.vi"("error in (no error)"=w1183, "Position (0 units)"=w1175, "Axis (1)"=w1176, "VISA resource name"=w1184) -> ("error out"=w1182:errorcluster, "VISA resource name out"=w1181:refnum<visa-resource-name>)  [unwired: 2 in]
      }
      frame "abs" {
        n650 = Dequeue Element(queue=w1192) -> ()  [unwired: 2 in, 4 out]
        n651 = Match Pattern(string=w1199, regular expression=":") -> (before substring=w1200:string, after substring=w1188:string)  [unwired: 1 in, 2 out]
        n652 = Match Pattern(string=w1188, regular expression=":") -> (before substring=w1187:string, after substring=w1186:string)  [unwired: 1 in, 2 out]
        n653 = Decimal String To Number(string=w1200) -> (number=w1196:i32)  [unwired: 2 in, 1 out]
        n654 = Fract/Exp String To Number(string=w1187) -> (number=w1185:dbl)  [unwired: 3 in, 1 out]
        n655 = call "Move Absolute.vi"("error in (no error)"=w1198, "Position (0 units)"=w1185, "Axis (1)"=w1196, "VISA resource name"=w1197) -> ("error out"=w1194:errorcluster, "VISA resource name out"=w1195:refnum<visa-resource-name>)  [unwired: 2 in]
        n656 = case shown="\"wait\"" w1186 {
          tunnel: w1196 -> [_ w1208]
          tunnel: w1195 -> [w1203 w1213]
          tunnel: w1194 -> [w1202 w1212]
          tunnel: [w1203 w1205] -> w1193
          tunnel: [w1202 w1211] -> w1191
          tunnel: w1190 -> [_ w1210]
          frame "", Default {
          }
          frame "wait" {
            n657 = while {
              tunnel: w1208 -> [w1222]
              shift-right: [w1219] -> w1207
              shift-left: w1213 -> [w1221]
              shift-right: [w1218] -> w1206
              shift-left: w1212 -> [w1220]
              stop <- w1217 stop-if-true
              n658 = call "Get Axis Motion Status.vi"("error in (no error)"=w1220, "Axis (1)"=w1222, "VISA resource name"=w1221) -> ("error out"=w1218:errorcluster, "Motion Done"=w1217:bool, "VISA resource name out"=w1219:refnum<visa-resource-name>)  [unwired: 2 in]
            }
            n659 = flat-sequence {
              tunnel: w1207 -> [w1216]
              tunnel: w1206 -> [w1215]
              tunnel: [w1216] -> w1205
              tunnel: [w1215] -> w1204
              frame #0 {
                n660 = Wait (ms)(milliseconds to wait=u32 1000) -> ()  [unwired: 1 out]
              }
            }
            n661 = Enqueue Element(queue=w1210, element="done", error in (no error)=w1204) -> (error out=w1211:errorcluster)  [unwired: 1 in, 2 out]
          }
        }
      }
      frame "suspend" {
        n662 = Dequeue Element(queue=w1226) -> ()  [unwired: 2 in, 4 out]
      }
      frame "release" {
        n663 = Dequeue Element(queue=w1227) -> ()  [unwired: 2 in, 4 out]
        n664 = call "Close.vi"("VISA resource name"=w1230) -> ("error out"=w1229:errorcluster)  [unwired: 10 in]
      }
      frame "close" {
        n665 = Release Queue(queue=w1234) -> ()  [unwired: 2 in, 3 out]
      }
      frame "init" {
        n666 = Dequeue Element(queue=w1239) -> ()  [unwired: 2 in, 4 out]
        n667 = flat-sequence {
          tunnel: [w1242] -> w1236
          tunnel: [w1241] -> w1235
          tunnel: [w1246] -> w1237
          tunnel: [w1247] -> w1238
          tunnel: w1236 -> [w1247]
          tunnel: w1235 -> [w1246]
          frame #0 {
            n668 = local write "ESP_con?"(FALSE ("ESP_con?")) -> ()
          }
          frame #1 {
            n669 = call "Initialize.vi"("VISA resource name"="ESP301 VISA", "Serial Link (RS232)"=enum16{"RS232", "USB"}."USB") -> ("VISA resource name out"=w1242:refnum<visa-resource-name>, "error out"=w1241:errorcluster)  [unwired: 7 in]
          }
          frame #2 {
            n670 = local write "ESP_con?"(TRUE ("ESP_con?")) -> ()
          }
        }
      }
    }
    "error out" <- w1156
  }
  n671 = while {
    tunnel: w3 -> [w1256]
    shift-right: [w1254] -> _
    shift-left: _ -> [w1252]
    shift-right: [w1253] -> _
    shift-left: _ -> [w1251]
    shift-right: [w1249] -> _
    shift-left: 0 -> [w1250]
    tunnel: w2 -> [w1248]
    stop <- w1255 stop-if-true
    # "manip"
    n672 = Preview Queue Element(queue=w1256, timeout in ms (-1)=w1250) -> (queue out=w1259:refnum<queue>, element=w1260:string)  [unwired: 1 in, 2 out]
    n673 = Match Pattern(string=w1260, regular expression=":") -> (before substring=w1258:string, after substring=w1257:string)  [unwired: 1 in, 2 out]
    n674 = case shown="\"idle\", Default" w1258 {
      tunnel: w1259 -> [_ w1272 w1299 w1326 w1330 w1339 w1344]
      tunnel: w1257 -> [_ _ w1286 _ _ _ _]
      tunnel: [_ _ _ _ _ TRUE _] -> w1255
      tunnel: [w1266 w1274 w1278 w1328 refnum<k5> refnum ("gateway_connection out") w1337 w1343] -> w1254
      tunnel: [w1265 w1273 w1280 w1327 w1332 w1336 w1342] -> w1253
      tunnel: w1252 -> [w1268 w1276 w1302 w1328 w1334 w1337 _]
      tunnel: w1251 -> [w1267 w1275 w1301 w1327 _ w1336 _]
      tunnel: [_ _ _ -1 _ _ _] -> w1249
      tunnel: w1248 -> [_ _ w1277 _ _ _ _]
      frame "idle", Default {
        n675 = call "sp_manip_get_axis_status.vi"("error in"=w1267, "gateway_connection"=w1268) -> ("error out"=w1265:errorcluster, "axis_out"=w1264:T9, "gateway_connection out"=w1266:refnum<k5>)  [unwired: 5 in, 2 out]
        n676 = for {
          tunnel: w1264 -> [w1271] mode=indexing
          tunnel: [w1270] -> w1263 mode=indexing
          tunnel: [w1269] -> w1262 mode=indexing
          n677 = Unbundle By Name(w1271) -> ("Axis_Position"=w1270:dbl, "moving"=w1269:bool)
        }
        "moving?" <- w1262
        n678 = local write "pos"(w1263) -> ()
      }
      frame "stop" {
        n679 = Dequeue Element(queue=w1272) -> ()  [unwired: 2 in, 4 out]
        n680 = call "sp_manip_abort.vi"("error in"=w1275, "gateway_connection"=w1276) -> ("error out"=w1273:errorcluster, "gateway_connection out"=w1274:refnum<k5>)  [unwired: 6 in, 2 out]
      }
      frame "relative" {
        n681 = Dequeue Element(queue=w1299) -> ()  [unwired: 2 in, 4 out]
        n682 = Match Pattern(string=w1286, regular expression=":") -> (before substring=w1285:string, after substring=w1284:string)  [unwired: 1 in, 2 out]
        n683 = Equal?(x=w1284, y="wait") -> (x = y?=w1282:bool)
        n684 = call "sp_manip_get_axis_status.vi"("error in"=w1301, "gateway_connection"=w1302) -> ("error out"=w1304:errorcluster, "axis_out"=w1291:T9, "gateway_connection out"=w1303:refnum<k5>)  [unwired: 5 in, 2 out]
        n685 = Scan From String(format string="%g_%g_%g_%g_%g_%g", input string=w1285) -> (output 1=w1298:dbl, output 2=w1297:dbl, output 3=w1296:dbl, output 4=w1295:dbl, output 5=w1294:dbl, output 6=w1293:dbl)  [unwired: 8 in, 3 out]
        n686 = for {
          tunnel: w1291 -> [w1325] mode=indexing
          tunnel: [w1324] -> w1289 mode=indexing
          tunnel: [w1323] -> w1290 mode=indexing
          n687 = Unbundle By Name(w1325) -> ("Axis_Name"=w1324:string, "Axis_Position"=w1323:dbl)
        }
        n688 = Build Array(w1298, w1297, w1296, w1295, w1294, w1293) -> (w1292:dbl[])
        n689 = Add(x=w1290, y=w1292) -> (x+y=w1288:dbl[])
        n690 = call "sp_manip_start_move.vi"("error in"=w1304, "target positions"=w1288, "axis names"=w1289, "gateway_connection"=w1303) -> ("error out"=w1281:errorcluster, "gateway_connection out"=w1279:refnum<k5>)  [unwired: 4 in, 2 out]
        n691 = case shown="True" w1282 {
          tunnel: w1281 -> [w1305 w1312]
          tunnel: [w1305 w1308] -> w1280
          tunnel: w1279 -> [w1306 w1313]
          tunnel: [w1306 w1311] -> w1278
          tunnel: w1277 -> [_ w1307]
          frame False {
          }
          frame True {
            n692 = while {
              tunnel: w1313 -> [w1317]
              tunnel: w1312 -> [w1316]
              tunnel: [w1315] -> w1311
              tunnel: [w1314] -> w1309
              stop <- w1318 continue-if-true
              n693 = call "sp_manip_get_axis_status.vi"("error in"=w1316, "gateway_connection"=w1317) -> ("error out"=w1314:errorcluster, "axis_out"=w1320:T9, "gateway_connection out"=w1315:refnum<k5>)  [unwired: 5 in, 2 out]
              n694 = for {
                tunnel: w1320 -> [w1322] mode=indexing
                tunnel: [w1321] -> w1319 mode=indexing
                n695 = Unbundle By Name(w1322) -> ("moving"=w1321:bool)
              }
              n696 = Or Array Elements(Boolean array=w1319) -> (logical OR=w1318:bool)
            }
            n697 = Enqueue Element(queue=w1307, element="done", error in (no error)=w1309) -> (error out=w1308:errorcluster)  [unwired: 1 in, 2 out]
          }
        }
      }
      frame "suspend" {
        n698 = Dequeue Element(queue=w1326) -> ()  [unwired: 2 in, 4 out]
      }
      frame "release" {
        n699 = Dequeue Element(queue=w1330) -> ()  [unwired: 2 in, 4 out]
        n700 = call "sp_manip_disconnect.vi"("gateway_connection"=w1334) -> ("error out"=w1333:errorcluster, "gateway_connection_out"=w1335:refnum<k5>)  [unwired: 7 in, 2 out]
        n701 = call "tcp_gateway_close_connection.vi"("error in"=w1333, "server_connection"=w1335) -> ("error out"=w1332:errorcluster)  [unwired: 5 in]
      }
      frame "close" {
        n702 = Release Queue(queue=w1339) -> ()  [unwired: 2 in, 3 out]
      }
      frame "init" {
        n703 = Dequeue Element(queue=w1344) -> ()  [unwired: 2 in, 4 out]
        n704 = flat-sequence {
          tunnel: [w1347] -> w1341
          tunnel: [w1346] -> w1340
          tunnel: [w1357] -> w1342
          tunnel: [w1358] -> w1343
          tunnel: w1341 -> [w1358]
          tunnel: w1340 -> [w1357]
          frame #0 {
            n705 = local write "manip_con?"(FALSE ("manip_con?")) -> ()
          }
          frame #1 {
            n706 = call "tcp_gateway_open_connection.vi"() -> ("gateway_connection"=w1350:refnum<k5>, "error out"=w1349:errorcluster)  [unwired: 5 in, 3 out]
            n707 = call "sp_manip_connect.vi"("error in"=w1349, "gateway_connection"=w1350) -> ("error out"=w1346:errorcluster, "axis_out"=w1348:T9, "gateway_connection out"=w1347:refnum<k5>)  [unwired: 5 in, 2 out]
            n708 = for {
              tunnel: w1348 -> [w1355] mode=indexing
              tunnel: [w1354] -> w1351 mode=indexing
              tunnel: [w1353] -> w1352 mode=indexing
              n709 = Unbundle By Name(w1355) -> ("Axis_Name"=w1354:string, "Axis_Position"=w1353:dbl)
            }
            "axis" <- w1351
            "pos" <- w1352
            n710 = local write "dest"(w1352) -> ()
          }
          frame #2 {
            n711 = local write "manip_con?"(TRUE ("manip_con?")) -> ()
          }
        }
      }
    }
    "error out 2" <- w1253
  }
  n712 = while {
    tunnel: w24 -> [w1369]
    shift-right: [w1366] -> _
    shift-left: 0 -> [w1367]
    shift-right: [w1365] -> _
    shift-left: _ -> [w1364]
    shift-right: [w1363] -> _
    shift-left: _ -> [w1362]
    shift-right: [w1361] -> _
    shift-left: u32 0 ("pHandle") -> [w1360]
    tunnel: string[] ["Kinetic Energy", "Pass Energy", "Coil Current", "Work Function", "Detector Voltage", "Screen Voltage", "Conversion Voltage", "Focus Displacement 1", "Focus Displacement 2"] -> [w1359]
    stop <- w1368 stop-if-true
    # "phoib"
    n713 = Preview Queue Element(queue=w1369, timeout in ms (-1)=w1367) -> (queue out=w1372:refnum<queue>, element=w1373:string)  [unwired: 1 in, 2 out]
    n714 = Match Pattern(string=w1373, regular expression=":") -> (before substring=w1371:string, after substring=w1370:string)  [unwired: 1 in, 2 out]
    n715 = case shown="\"idle\", Default" w1371 {
      tunnel: w1372 -> [_ w1426 w1442 w1458 w1472 w1476 w1482]
      tunnel: w1370 -> [_ _ _ _ _ _ _]
      tunnel: [_ _ _ _ TRUE _ _] -> w1368
      tunnel: [_ _ _ _ _ -1 _] -> w1366
      tunnel: [w1383 w1428 w1445 w1456 w1470 w1475 w1479] -> w1365
      tunnel: w1364 -> [w1394 w1417 w1447 w1457 w1470 w1475 _]
      tunnel: [w1382 w1427 w1444 w1455 w1468 w1473 w1478] -> w1363
      tunnel: w1362 -> [w1392 w1416 w1446 _ w1468 w1473 _]
      tunnel: [w1380 w1414 w1443 w1454 w1469 w1474 w1481] -> w1361
      tunnel: w1360 -> [w1380 w1414 w1443 w1453 w1469 w1474 _]
      tunnel: w1359 -> [w1381 w1407 _ _ _ _ _]
      frame "idle", Default {
        n716 = call "SL2_AD_DLL_Phoibos_GetDeviceState.vi"("dll_path"=w1394, "pHandle_in"=w1380, "dev_type"=DEF_dev_type."devA (analyzer)", "error in"=w1392) -> ("path out"=w1379:path, "state"=→"state":T4, "error out"=w1378:errorcluster)  [unwired: 2 in]
        n717 = for {
          tunnel: w1380 -> [w1401]
          tunnel: w1381 -> [w1399] mode=indexing
          tunnel: [w1398] -> w1391 mode=indexing
          tunnel: [w1397] -> w1383
          shift-right: [w1396] -> w1382
          shift-left: w1378 -> [w1400]
          tunnel: w1379 -> [w1395]
          n718 = call "SL2_AD_DLL_Phoibos_GetVoltage.vi"("error in"=w1400, "voltage_name"=w1399, "pHandle"=w1401, "dll path in"=w1395) -> ("error out"=w1396:errorcluster, "value"=w1398:dbl, "dll path out"=w1397:path)  [unwired: 3 in]
        }
        n719 = Index Array(array=w1391) -> (element #1=→"phoib_I_1":dbl, element #2=→"phoib_I_2":dbl, element #3=→"phoib_I_3":dbl, element #4=→"phoib_I_4":dbl, element #5=→"phoib_I_5":dbl, element #6=→"phoib_I_6":dbl, element #7=→"phoib_I_7":dbl, element #8=→"phoib_I_8":dbl, element #9=→"phoib_I_9":dbl)  [unwired: 9 in]
      }
      frame "set" {
        n720 = Dequeue Element(queue=w1426) -> ()  [unwired: 2 in, 4 out]
        n721 = Multiply(x="VoltageRange", y=13) -> (x*y=w1423:i32)
        n722 = Add(x="Mode", y=w1423) -> (x+y=w1420:i32)
        n723 = Index Array(array=u32[] [251749632, 251749633, 251749634, 251749635, 251749636, 251749637, 251749638, 251749639, 251749640, 251749641, 251749642, 251749643, 251749644, 251749645, 251749646, 251749647, 251749648, 251749649, 251749650, 251749651, 251749652, 251749653, 251749654, 251749655, 251749656, 251749657, 251749658, 251749659, 251749660, 251749661, 251749662, 251749663, 251749664, 251749665, 251749666, 251749667, 251749668, 251749669, 251749670, 251749671, 251749672, 251749673, 251749674, 251749675, 251749676, 251749677, 251749678, 251749679, 251749680, 251749681, 251749682, 251749683, 251749684, 251749685, 251749686, 251749687, 251749688, 251749689, 251749690, 251749691, 251749692, 251749693, 251749694, 251749695, 251749696] ("modeIDs"), index=w1420) -> (element=w1418:u32)
        n724 = Build Array("phoib_I_1s", "phoib_I_2s", "phoib_I_3s", "phoib_I_4s", "phoib_I_5s", "phoib_I_6s", "phoib_I_7s", "phoib_I_8s", "phoib_I_9s") -> (w1406:dbl[])
        n725 = call "SL2_AD_DLL_Phoibos_SetDeviceMode.vi"("pHandle"=w1414, "error in"=w1416, "value"=w1418, "dev_type"=DEF_dev_type."devA (analyzer)", "dll path in"=w1417) -> ("error out"=w1405:errorcluster, "dll path out"=w1415:path)  [unwired: 4 in]
        n726 = for {
          tunnel: w1414 -> [w1434]
          shift-right: [w1441] -> w1428
          shift-left: w1415 -> [w1438]
          tunnel: w1407 -> [w1433] mode=indexing
          tunnel: w1406 -> [w1432] mode=indexing
          shift-right: [w1440] -> w1427
          shift-left: w1405 -> [w1436]
          n727 = call "SL2_AD_DLL_Phoibos_GetVoltageRange.vi"("error in"=w1436, "voltage_name"=w1433, "pHandle"=w1434, "dll path in"=w1438) -> ("error out"=w1435:errorcluster, "min"=w1430:dbl, "max"=w1431:dbl, "dll path out"=w1437:path)  [unwired: 2 in]
          n728 = In Range and Coerce(upper limit=w1431, x=w1432, lower limit=w1430) -> (coerced(x)=w1429:dbl)  [unwired: 1 out]
          n729 = call "SL2_AD_DLL_Phoibos_SetVoltage.vi"("commit"=TRUE, "pHandle"=w1434, "error in"=w1435, "value"=w1429, "voltageName"=w1433, "dll path in"=w1437) -> ("error out"=w1440:errorcluster, "dll path out"=w1441:path)  [unwired: 3 in]
        }
      }
      frame "standby" {
        w1448 = T4 0 items=["Off"=-1, "Standby"=0, "On"=1] ("state")
        n730 = Dequeue Element(queue=w1442) -> ()  [unwired: 2 in, 4 out]
        n731 = call "SL2_AD_DLL_Phoibos_SetDeviceState.vi"("pHandle_in"=w1443, "error in"=w1446, "state"=w1448, "dev_type"=DEF_dev_type."devA (analyzer)", "dll_path"=w1447) -> ("error out"=w1444:errorcluster, "path out"=w1445:path)  [unwired: 2 in]
      }
      frame "release" {
        n732 = Dequeue Element(queue=w1458) -> ()  [unwired: 2 in, 4 out]
        n733 = flat-sequence {
          tunnel: w1457 -> [w1459]
          tunnel: w1453 -> [w1460]
          tunnel: [w1463] -> w1452
          tunnel: [w1462] -> w1451
          tunnel: [u32 0] -> w1450
          tunnel: [w1465] -> w1454
          tunnel: [w1466] -> w1455
          tunnel: [w1467] -> w1456
          tunnel: w1452 -> [w1467]
          tunnel: w1451 -> [w1466]
          tunnel: w1450 -> [w1465]
          frame #0 {
            n734 = call "SL2_AD_DLL_Phoibos_Shutdown.vi"("pHandle"=w1460, "dll path in"=w1459) -> ("error out"=w1462:errorcluster, "dll path out"=w1463:path)  [unwired: 4 in]
          }
          frame #1 {
            n735 = local write "phoib_con?"(FALSE ("phoib_con?")) -> ()
          }
        }
      }
      frame "close" {
        n736 = Release Queue(queue=w1472) -> ()  [unwired: 2 in, 3 out]
      }
      frame "suspend" {
        n737 = Dequeue Element(queue=w1476) -> ()  [unwired: 2 in, 4 out]
      }
      frame "init" {
        n738 = Dequeue Element(queue=w1482) -> ()  [unwired: 2 in, 4 out]
        n739 = flat-sequence {
          tunnel: [w1489] -> w1480
          tunnel: [w1485] -> w1479
          tunnel: [w1484] -> w1478
          tunnel: [w1497] -> w1481
          tunnel: w1480 -> [w1497]
          frame #0 {
            n740 = local write "phoib_con?"(FALSE ("phoib_con?")) -> ()
          }
          frame #1 {
            w1488 = DEF_dev_type."devA (analyzer)" ("dev_type")
            n741 = call "GetSL2AD_VI_dllPath.vi"() -> ("error"=w1492:errorcluster, "Path"=w1493:path)  [unwired: 9 in, 1 out]
            n742 = call "SL2_AD_DLL_List_Devices.vi"("error in"=w1492, "dev_type"=w1488, "dll path in"=w1493) -> ("error out"=w1486:errorcluster, "devices"=w1495:string[], "dll path out"=w1487:path)  [unwired: 2 in]
            n743 = Index Array(array=w1495) -> (element=w1494:string)  [unwired: 1 in]
            n744 = call "SL2_AD_DLL_Phoibos_Initialize.vi"("error in"=w1486, "analyzerId"=w1494, "dll_path"=w1487) -> ("error out"=w1490:errorcluster, "pHandle"=w1489:u32, "path out"=w1491:path)  [unwired: 2 in]
            n745 = call "SL2_AD_DLL_Phoibos_ListDeviceModes.vi"("dll path in"=w1491, "dev_type"=w1488, "pHandle"=w1489, "error in"=w1490) -> ("dll path out"=w1485:path, "error out"=w1484:errorcluster)  [unwired: 1 in, 2 out]
          }
          frame #2 {
            n746 = local write "phoib_con?"(TRUE ("phoib_con?")) -> ()
          }
        }
      }
    }
    "phoib_error" <- w1363
  }
